vi "Update Registry.vi"() -> ()   [LabVIEW 2014]
uses:
  TypeDef/state.ctl
  TypeDef/Qmessage.ctl
  <vilib>/Utility/config.llb/Read Key (Path).vi
  <vilib>/Utility/file.llb/Read From Spreadsheet File (string).vi
  <vilib>/Utility/config.llb/Write Key (Path).vi
  <vilib>/Utility/config.llb/Read Key (String).vi
  <vilib>/Utility/config.llb/NI_LVConfig.lvlib
panel:
  out "Internal State":T1
  out "Date":string
  out "Time":string
  out "Status bar":string
  in  "Build New Config":bool
  in  "Tab Control":T2(tab)
  in  "Changed?":bool[](array[boolean])
  in  "Current Configuration":string[](array[string])
  in  "Component Name":string[](array[string])
  in  "New Configuration":string[](array[string])
  in  "Changed? 2":bool[](array[boolean])
  in  "Current Configuration 2":string[](array[string])
  in  "Component Name 2":string[](array[string])
  in  "New Configuration 2":string[](array[string])
  in  "Changed? 3":bool[](array[boolean])
  in  "Current Configuration 3":string[](array[string])
  in  "Component Name 3":string[](array[string])
  in  "New Configuration 3":string[](array[string])
  in  "Changed? 4":bool[](array[boolean])
  in  "Current Configuration 4":string[](array[string])
  in  "Component Name 4":string[](array[string])
  in  "New Configuration 4":string[](array[string])
  in  "Changed? 5":bool[](array[boolean])
  in  "Current Configuration 5":string[](array[string])
  in  "Component Name 5":string[](array[string])
  in  "New Configuration 5":string[](array[string])
  in  "Changed? 6":bool[](array[boolean])
  in  "Current Configuration 6":string[](array[string])
  in  "Component Name 6":string[](array[string])
  in  "New Configuration 6":string[](array[string])
  in  "Changed? 7":bool[](array[boolean])
  in  "Current Configuration 7":string[](array[string])
  in  "Component Name 7":string[](array[string])
  in  "New Configuration 7":string[](array[string])
  in  "Changed? 8":bool[](array[boolean])
  in  "Current Configuration 8":string[](array[string])
  in  "Component Name 8":string[](array[string])
  in  "New Configuration 8":string[](array[string])
  in  "Changed? 9":bool[](array[boolean])
  in  "Current Configuration 9":string[](array[string])
  in  "Component Name 9":string[](array[string])
  in  "New Configuration 9":string[](array[string])
  in  "Changed? 10":bool[](array[boolean])
  in  "Current Configuration 10":string[](array[string])
  in  "Component Name 10":string[](array[string])
  in  "New Configuration 10":string[](array[string])
  out "ini file path":path
  in  "variation sheet":path caption="Variation Sheet (*.ini)"
  in  "Push":bool
  in  "Help Button":bool
  in  "Run":bool
  in  "Initialize":bool
  in  "Register":bool
  in  "Add comment":bool
  in  "View":bool
  in  "tdms path":path caption="Variation Registry (*.tdms)"
  in  "Config Path":path caption="Config File (*.csv)"
  in  "Exit":bool
  # "Update Registry"
  # "New Configuration"
  # "Component Name"
  # "Current Configuration"
  # "New Configuration"
  # "Component Name"
  # "Current Configuration"
  # "New Configuration"
  # "Component Name"
  # "Current Configuration"
  # "New Configuration"
  # "Component Name"
  # "Current Configuration"
  # "New Configuration"
  # "Component Name"
  # "Current Configuration"
  # "New Configuration"
  # "Component Name"
  # "Current Configuration"
  # "New Configuration"
  # "Component Name"
  # "Current Configuration"
  # "New Configuration"
  # "Component Name"
  # "Current Configuration"
  # "New Configuration"
  # "Component Name"
  # "Current Configuration"
  # "New Configuration"
  # "Component Name"
  # "Current Configuration"
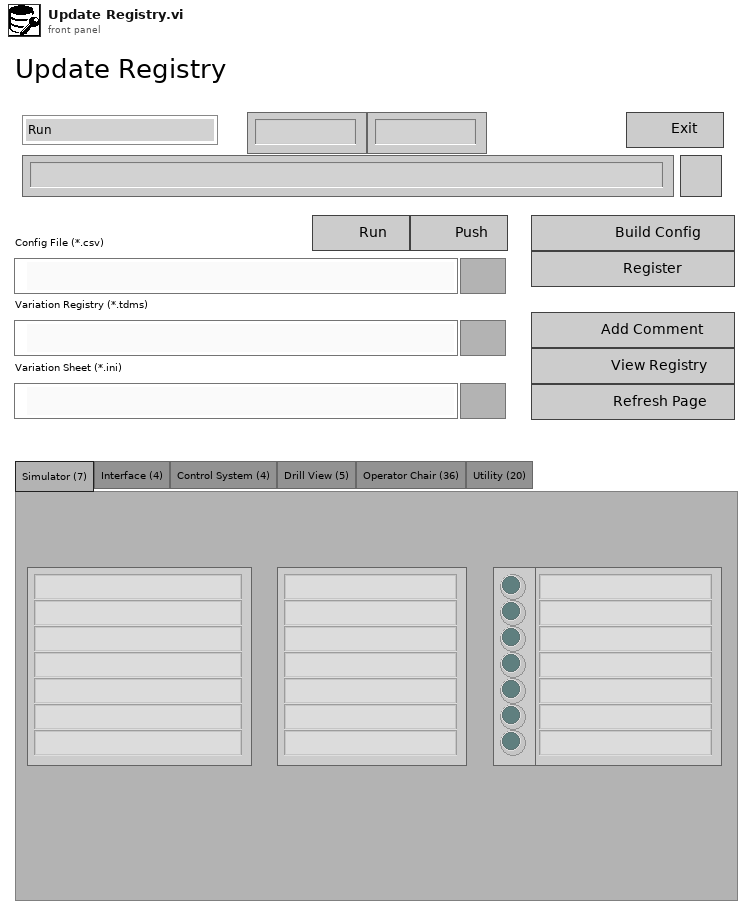
[diagram p1: front panel]
types:
  T1 = typedef "state.ctl" = enum16{"Run", "Initialize 1", "Initialize 2", "Read config file", "Read TDMS", "Config file Error", "Idle", "Update Comp Names", "Update Current Versions", "Make new configuration", "Register Change", "View Registry", "Add Comment", "No New Update", "Check current versions", "Read ini file", "Write ini file", "Read Variation Sheet", "Search and write current versions", "Close", "Update New Config", "Check ini file"}
  T2 = enum32{"Page 1", "Page 2", "Page 3", "Page 4", "Page 5", "Page 6", "Page 7", "Page 8", "Page 9", "Page 10"}
  T3 = cluster{"Folder Path containing version information":path, "File name (including .ini)":path, "Section":string}
  T4 = typedef "Qmessage.ctl" = cluster{"state":T1, "data":variant}
  T5 = cluster{"path":path, "This VI":refnum<vi>, "Level of Application":u8}
  T6 = enum32{"invalid app kind", "Development System", "Run Time System", "Student Edition", "Embedded LabVIEW", "Evaluation", "Custom"}
  T7 = cluster{"Current Version":string[], "Comp Name":string[]}
  T8 = enum8{"Enabled", "Disabled", "Disabled and Grayed Out"}
  T9 = typedef "NI_LVConfig.lvlib/Config Data RefNum.ctl" = refnum<k1>
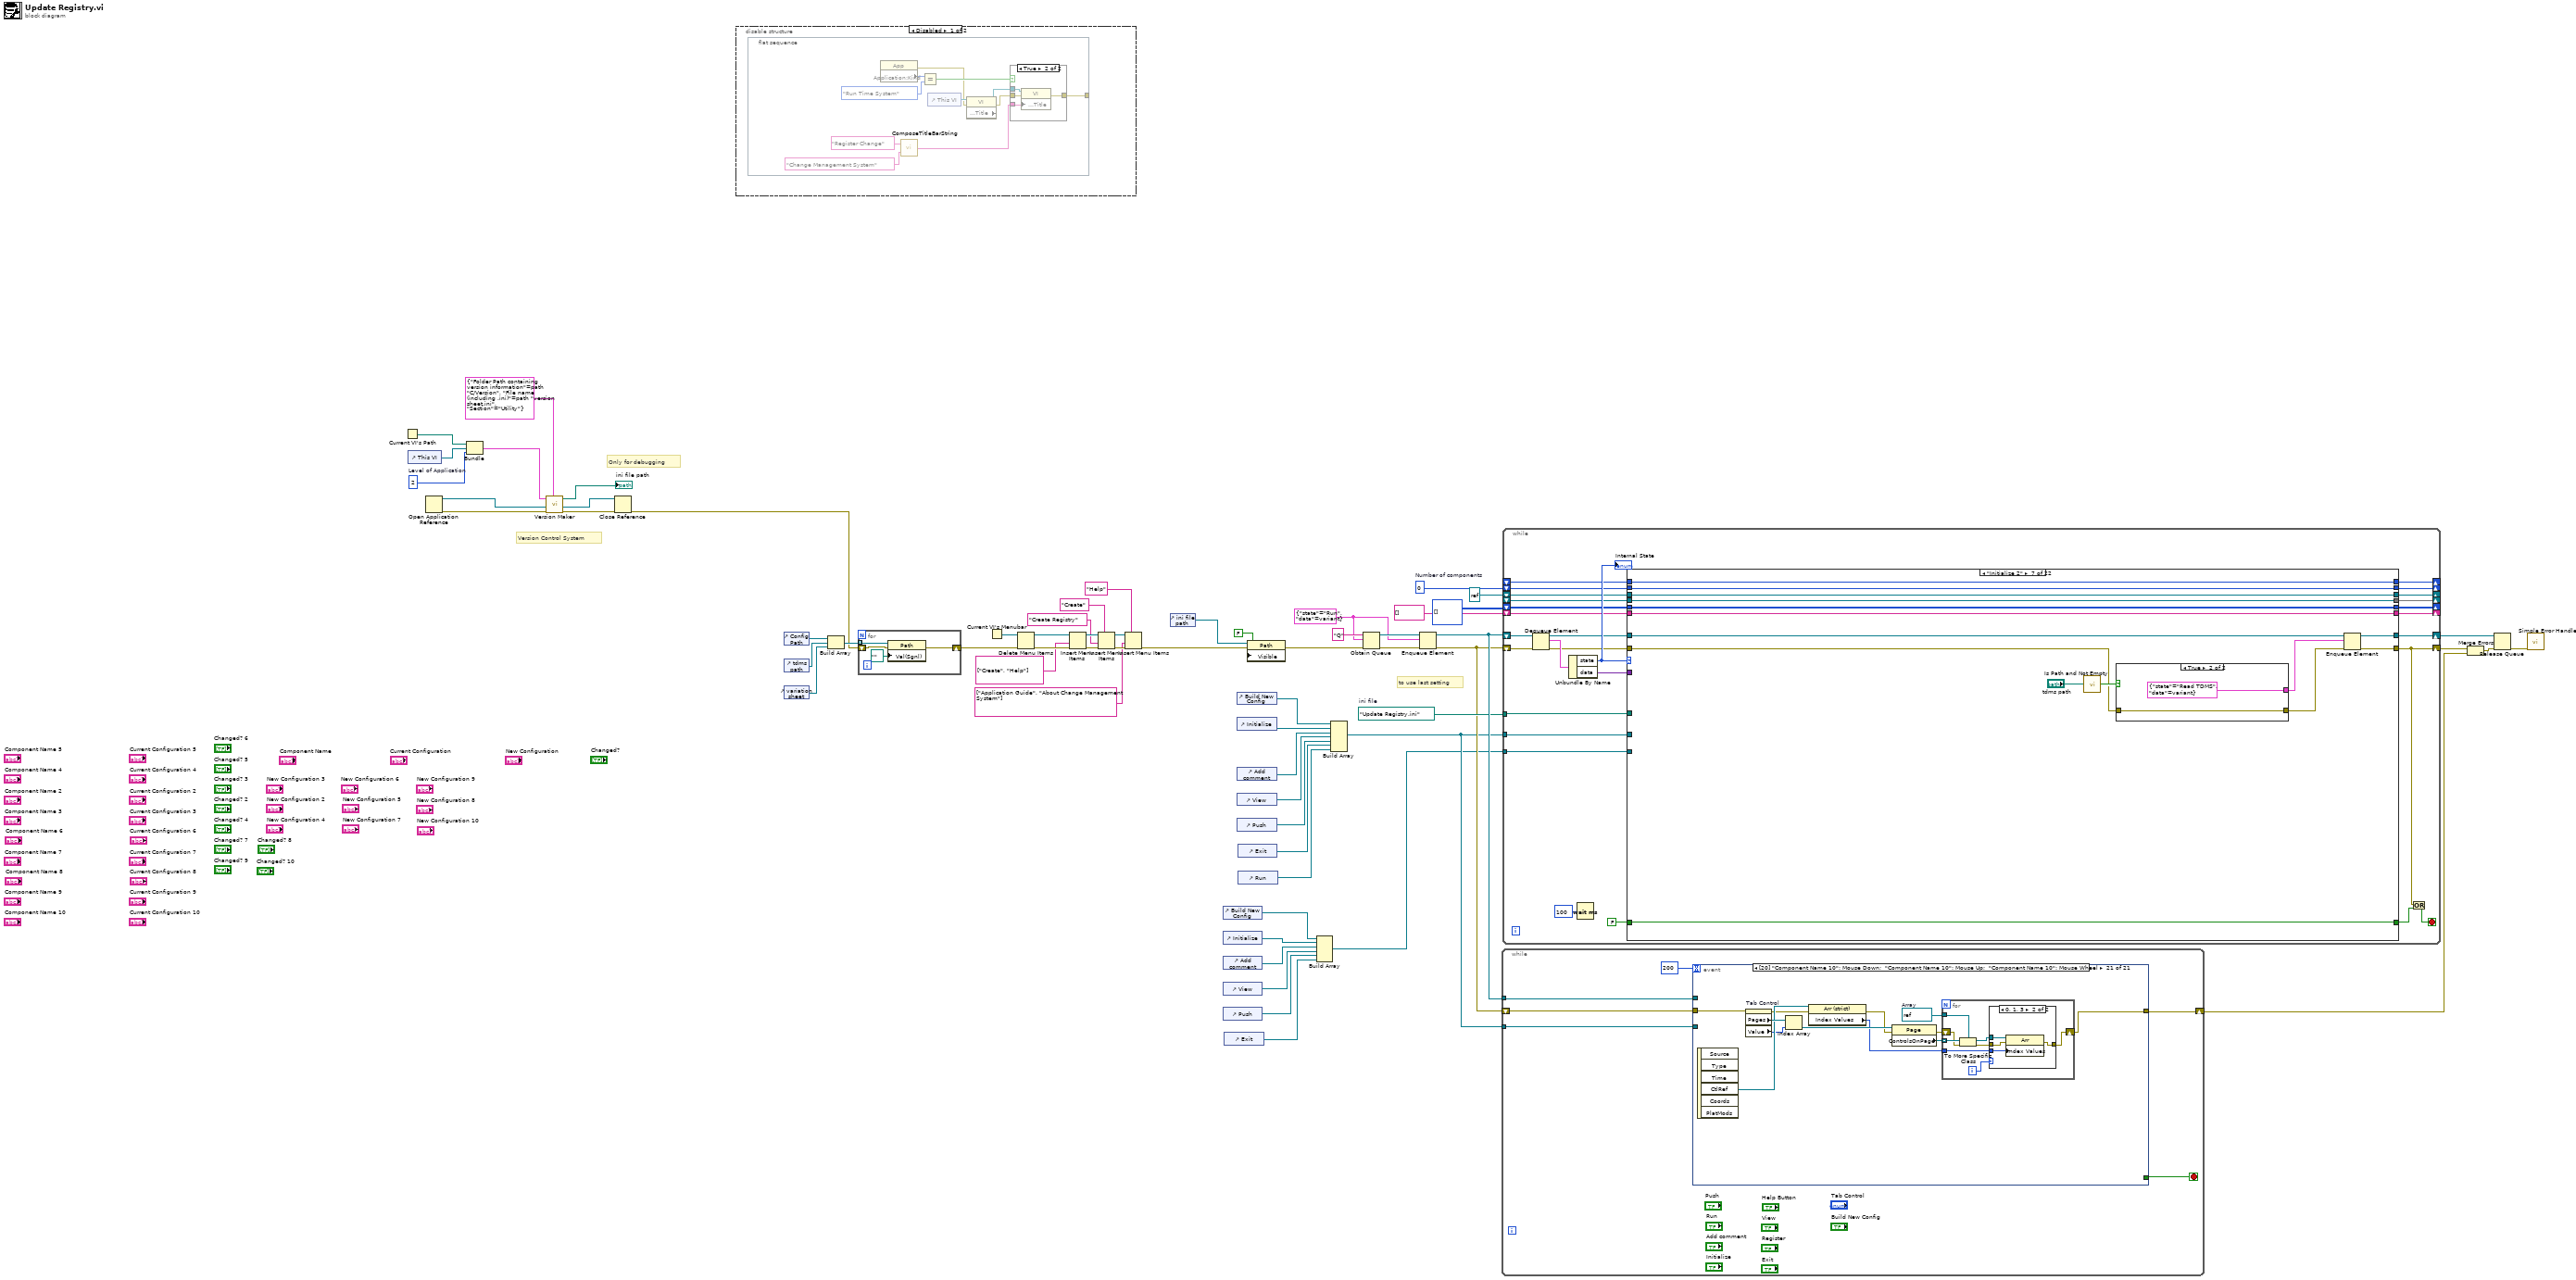
[diagram p0: block diagram]
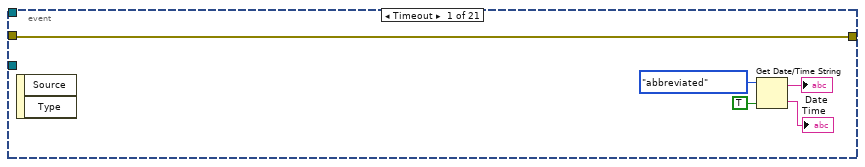
[diagram p4: hidden frame]
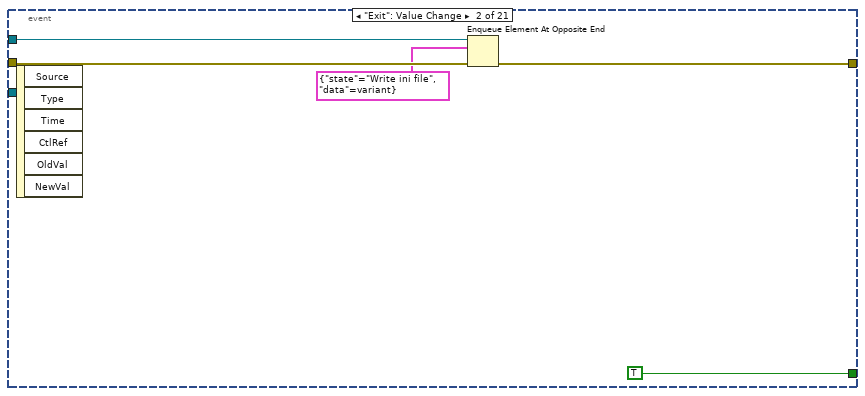
[diagram p5: hidden frame]
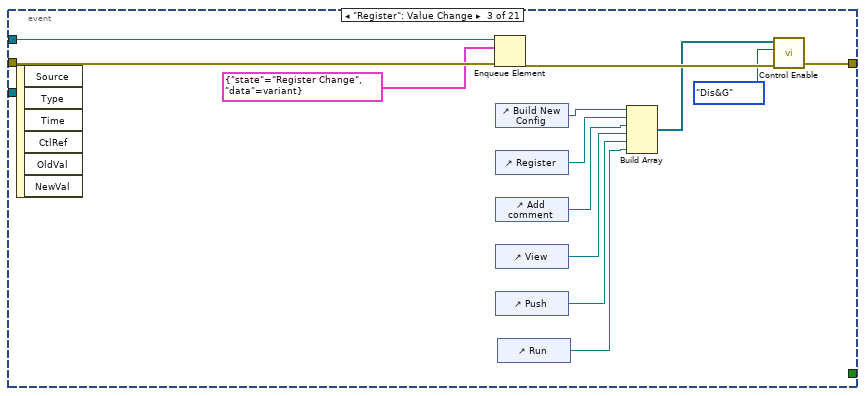
[diagram p6: hidden frame]
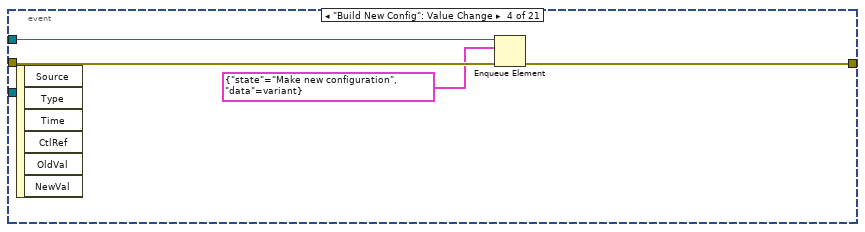
[diagram p7: hidden frame]
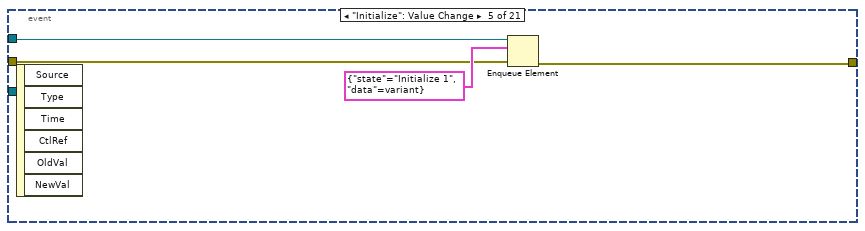
[diagram p8: hidden frame]
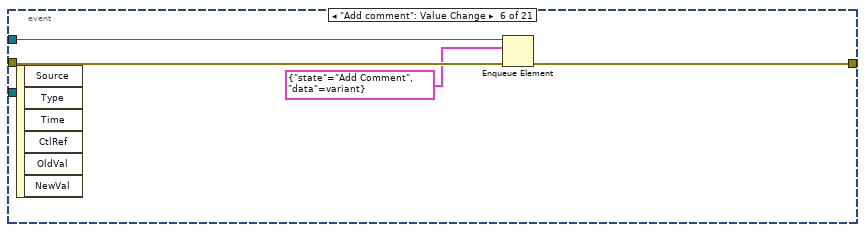
[diagram p9: hidden frame]
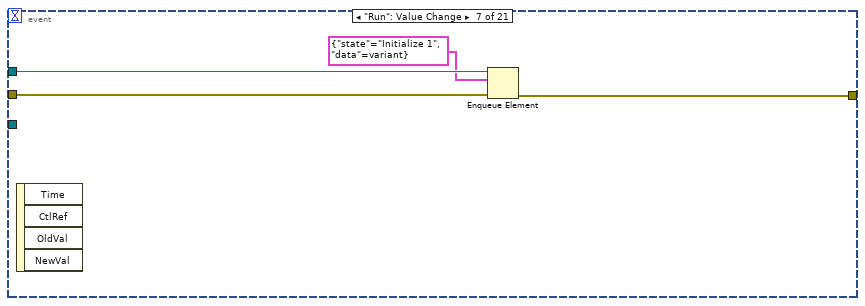
[diagram p10: hidden frame]
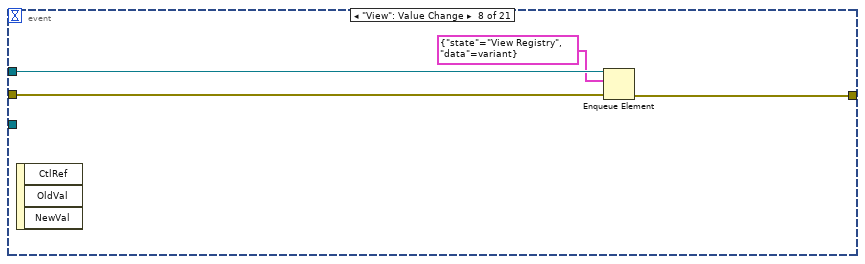
[diagram p11: hidden frame]
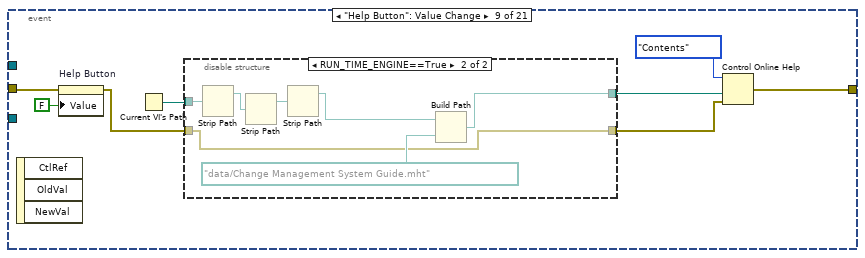
[diagram p12: hidden frame]
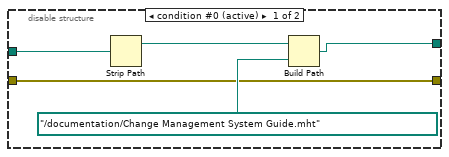
[diagram p13: hidden frame]
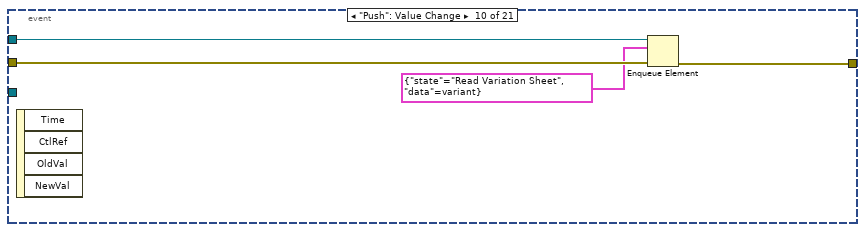
[diagram p14: hidden frame]
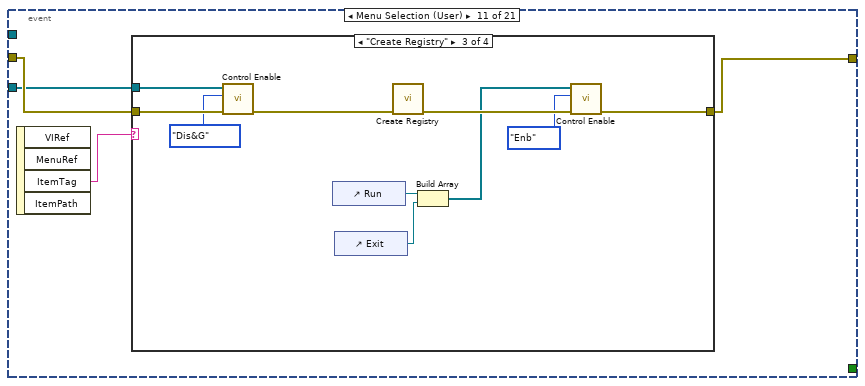
[diagram p15: hidden frame]
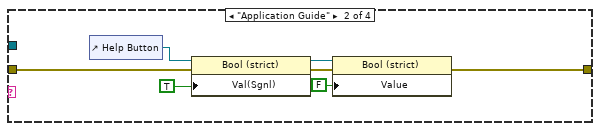
[diagram p17: hidden frame]
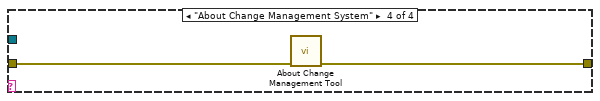
[diagram p18: hidden frame]
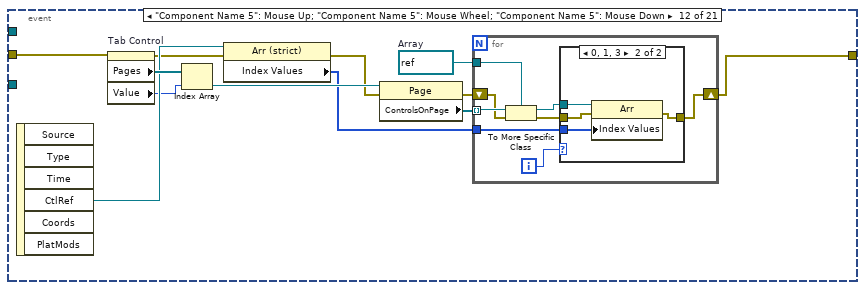
[diagram p19: hidden frame]
diagram:
  w44 = u8 2  # Level of Application
  w55 = path "Update Registry.ini"  # ini file
  w59 = 0  # Number of components
  w28 = T4 {"state"=enum."Run", "data"=variant} ("Cluster")
  # "to use last setting"
  # "Only for debugging"
  # "Version Control System"
  n1 = Current VI's Path() -> (path=w42:path)
  n2 = control-ref of="This VI"() -> (w43:refnum<vi>)
  n3 = Open Application Reference() -> (0:w54:errorcluster, 3:w50:refnum<vi>)  [unwired: 4 in]
  n4 = Bundle("path"=w42, "This VI"=w43, "Level of Application"=w44) -> (w45:T5)  [unwired: 1 in]
  n5 = call "Version Maker.vi"("Version Sheet Cluster"=T3 {"Folder Path containing version information"=path "C:/Version", "File name (including .ini)"=path "version sheet.ini", "Section"="Utility"}, "Error In"=w54, "Open Application Reference in"=w50, "VI Information"=w45) -> ("Error Out"=w53:errorcluster, "Open Application Reference out"=w49:refnum<vi>, "Standard Config Path"=→"ini file path":path)  [unwired: 4 in, 1 out]
  n6 = Close Reference(reference=w49, error in (no error)=w53) -> (error out=w22:errorcluster)
  n7 = disable-structure shown="Disabled" {
    frame Disabled {
      n8 = flat-sequence {
        tunnel: [w64] -> _
        frame #0 {
          n9 = property on="Property Node" class="App"() -> (error out=w66:errorcluster, "Application:Kind"=w72:T6)  [unwired: 2 in, 1 out]
          n10 = call "ComposeTitleBarString.vi"("ProjectName"="Change Management System" ("Application"), "Application"="Register Change") -> ("TitleBar"=w74:string)
          n11 = Equal?(x=w72, y=T6."Run Time System" ("Applikation:Typ")) -> (x = y?=w73:bool)
          n12 = control-ref of="This VI"() -> (w70:refnum<vi>)
          n13 = property on="Property Node" class="VI" props=["Front Panel.Title"](reference=w70, error in=w66) -> (reference out=w69:refnum<vi>, error out=w65:errorcluster)  [unwired: 1 out]
          n14 = case shown="True" w73 {
            tunnel: w74 -> [_ w79]
            tunnel: w69 -> [_ w78]
            tunnel: w65 -> [w75 w77]
            tunnel: [w75 w76] -> w64
            frame False {
            }
            frame True {
              n15 = property class="VI"(reference=w78, error in=w77, "Front Panel.Title"=w79) -> (error out=w76:errorcluster)  [unwired: 1 out]
            }
          }
        }
      }
    }
    frame Enabled {
    }
  }
  n16 = control-ref of="Config Path"() -> (w26:refnum<vi>)
  n17 = control-ref of="tdms path"() -> (w25:refnum<vi>)
  n18 = control-ref of="variation sheet"() -> (w24:refnum<vi>)
  n19 = Build Array(w26, w25, w24) -> (w23:refnum<vi>[])
  n20 = for {
    tunnel: w23 -> [w83] mode=indexing
    shift-right: [w81] -> w21
    shift-left: w22 -> [w80]
    n21 = property class="Path"(reference=w83, error in=w80, "Val(Sgnl)"=path "" ("Value (Signaling)")) -> (error out=w81:errorcluster)  [unwired: 1 out]
  }
  n22 = Current VI's Menubar() -> (w41:refnum<k9>)
  n23 = Delete Menu Items(6:w21, 9:w41) -> (0:w40:errorcluster, 3:w39:refnum<k9>)  [unwired: 2 in]
  n24 = Insert Menu Items(6:w40, 7:string[] ["Create", "Help"] ("item tags"), 9:w39) -> (0:w35:errorcluster, 3:w37:refnum<k9>)  [unwired: 3 in, 1 out]
  n25 = Insert Menu Items(5:"Create", 6:w35, 7:"Create Registry", 9:w37) -> (0:w34:errorcluster, 3:w33:refnum<k9>)  [unwired: 2 in, 1 out]
  n26 = Insert Menu Items(5:"Help", 6:w34, 7:string[] ["Application Guide", "About Change Management System"] ("item tags"), 9:w33) -> (0:w27:errorcluster)  [unwired: 2 in, 2 out]
  n27 = control-ref of="ini file path"() -> (w47:refnum<vi>)
  n28 = control-ref of="Build New Config"() -> (w2:refnum<vi>)
  n29 = control-ref of="Initialize"() -> (w3:refnum<vi>)
  n30 = control-ref of="Add comment"() -> (w5:refnum<vi>)
  n31 = control-ref of="View"() -> (w6:refnum<vi>)
  n32 = control-ref of="Push"() -> (w7:refnum<vi>)
  n33 = control-ref of="Exit"() -> (w4:refnum<vi>)
  n34 = control-ref of="Build New Config"() -> (w8:refnum<vi>)
  n35 = control-ref of="Initialize"() -> (w9:refnum<vi>)
  n36 = control-ref of="Add comment"() -> (w15:refnum<vi>)
  n37 = control-ref of="View"() -> (w14:refnum<vi>)
  n38 = control-ref of="Push"() -> (w13:refnum<vi>)
  n39 = control-ref of="Exit"() -> (w12:refnum<vi>)
  n40 = control-ref of="Run"() -> (w11:refnum<vi>)
  n41 = property class="Path"(reference=w47, error in=w27, "Visible"=FALSE) -> (error out=w48:errorcluster)  [unwired: 1 out]
  n42 = Build Array(w2, w3, w5, w6, w7, w4) -> (w1:refnum<vi>[])
  n43 = Build Array(w8, w9, w15, w14, w13, w12, w11) -> (w10:refnum<vi>[])
  n44 = Obtain Queue(name (unnamed)="Q", element data type=w28, error in (no error)=w48) -> (queue out=w63:refnum<queue>, error out=w58:errorcluster)  [unwired: 2 in, 1 out]
  n45 = Enqueue Element(queue=w63, element=w28, error in (no error)=w58) -> (queue out=w61:refnum<queue>, error out=w29:errorcluster)  [unwired: 1 in, 1 out]
  n46 = while {
    tunnel: w61 -> [w89]
    tunnel: w10 -> [w86]
    shift-right: [w85] -> w18
    shift-left: w29 -> [w87]
    stop <- w88 stop-if-true
    n47 = event shown="[20] \"Component Name 10\": Mouse Down;  \"Component Name 10\": Mouse Up;  \"Component Name 10\": Mouse Wheel" {
      selector: _ -> [_ _ _ _ _ _ _ _ _ _ _ _ _ _ _ _ _ _ _ _ _]
      dyn-events: _ -> [_ _ _ _ _ _ _ _ _ _ _ _ _ _ _ _ _ _ _ _ _]
      timeout: u32 200 ("milliseconds to wait") -> [_ _ _ _ _ _ _ _ _ _ _ _ _ _ _ _ _ _ _ _ _]
      tunnel: w89 -> [_ w99 w112 w116 w120 w124 w128 w132 _ w156 _ _ _ _ _ _ _ _ _ _ _]
      tunnel: [_ TRUE _ _ _ _ _ _ _ _ _ _ _ _ _ _ _ _ _ _ _] -> w88
      tunnel: [w90 w97 w109 w113 w119 w123 w127 w131 w139 w155 w158 w182 w207 w232 w257 w282 w307 w332 w357 w382 w407] -> w85
      tunnel: w87 -> [w90 w96 w111 w115 w117 w122 w126 w130 w135 w154 w159 w190 w215 w240 w265 w290 w315 w340 w365 w390 w415]
      tunnel: w86 -> [_ _ _ _ _ _ _ _ _ _ w157 _ _ _ _ _ _ _ _ _ _]
      event Timeout {
        n48 = event-data() -> ()  [unwired: 1 in, 2 out]
        n49 = Get Date/Time String(date format (0)=enum16{"short", "long", "abbreviated"}."abbreviated", want seconds? (F)=TRUE) -> (date string=→"Date":string, time string=→"Time":string)  [unwired: 1 in]
      }
      event "Exit": Value Change {
        n50 = event-data() -> ()  [unwired: 1 in, 6 out]
        n51 = Enqueue Element At Opposite End(queue=w99, element=T4 {"state"=enum."Write ini file", "data"=variant} ("Cluster"), error in (no error)=w96) -> (error out=w97:errorcluster)  [unwired: 1 in, 2 out]
      }
      event "Register": Value Change {
        n52 = event-data() -> ()  [unwired: 1 in, 6 out]
        n53 = Enqueue Element(queue=w112, element=T4 {"state"=enum."Register Change", "data"=variant} ("Cluster"), error in (no error)=w111) -> (error out=w108:errorcluster)  [unwired: 1 in, 2 out]
        n54 = control-ref of="Build New Config"() -> (w101:refnum<vi>)
        n55 = control-ref of="Register"() -> (w102:refnum<vi>)
        n56 = control-ref of="Add comment"() -> (w103:refnum<vi>)
        n57 = control-ref of="View"() -> (w104:refnum<vi>)
        n58 = control-ref of="Push"() -> (w105:refnum<vi>)
        n59 = control-ref of="Run"() -> (w106:refnum<vi>)
        n60 = Build Array(w101, w102, w103, w104, w105, w106) -> (w100:refnum<vi>[])
        n61 = call "Control Enable.vi"("error in (no error)"=w108, "Enum"=enum16{"Enb", "Dis", "Dis&G"}."Dis&G", "Reference Array"=w100) -> ("error out"=w109:errorcluster)  [unwired: 8 in]
      }
      event "Build New Config": Value Change {
        n62 = event-data() -> ()  [unwired: 1 in, 6 out]
        n63 = Enqueue Element(queue=w116, element=T4 {"state"=enum."Make new configuration", "data"=variant} ("Cluster"), error in (no error)=w115) -> (error out=w113:errorcluster)  [unwired: 1 in, 2 out]
      }
      event "Initialize": Value Change {
        n64 = event-data() -> ()  [unwired: 1 in, 6 out]
        n65 = Enqueue Element(queue=w120, element=T4 {"state"=enum."Initialize 1", "data"=variant} ("Cluster"), error in (no error)=w117) -> (error out=w119:errorcluster)  [unwired: 1 in, 2 out]
      }
      event "Add comment": Value Change {
        n66 = event-data() -> ()  [unwired: 1 in, 6 out]
        n67 = Enqueue Element(queue=w124, element=T4 {"state"=enum."Add Comment", "data"=variant} ("Cluster"), error in (no error)=w122) -> (error out=w123:errorcluster)  [unwired: 1 in, 2 out]
      }
      event "Run": Value Change {
        n68 = event-data() -> ()  [unwired: 1 in, 4 out]
        n69 = Enqueue Element(queue=w128, element=T4 {"state"=enum."Initialize 1", "data"=variant} ("Cluster"), error in (no error)=w126) -> (error out=w127:errorcluster)  [unwired: 1 in, 2 out]
      }
      event "View": Value Change {
        n70 = event-data() -> ()  [unwired: 1 in, 3 out]
        n71 = Enqueue Element(queue=w132, element=T4 {"state"=enum."View Registry", "data"=variant} ("Cluster"), error in (no error)=w130) -> (error out=w131:errorcluster)  [unwired: 1 in, 2 out]
      }
      event "Help Button": Value Change {
        n72 = event-data() -> ()  [unwired: 1 in, 3 out]
        n73 = property on="Help Button" class="Bool (strict)"(error in=w135, "Value"=FALSE ("Help Button")) -> (error out=w134:errorcluster)  [unwired: 1 in, 1 out]
        n74 = Current VI's Path() -> (path=w138:path)
        n75 = disable-structure shown="RUN_TIME_ENGINE==True" {
          disable-tunnel: w138 -> [w145 w152]
          disable-tunnel: [w142 w148] -> w137
          disable-tunnel: w134 -> [w141 w146]
          disable-tunnel: [w141 w146] -> w133
          frame condition #0 (active) {
            n76 = Strip Path(path=w145) -> (stripped path=w144:path)  [unwired: 1 out]
            n77 = Build Path(base path=w144, name or relative path=path "../documentation/Change Management System Guide.mht") -> (appended path=w142:path)
          }
          frame condition #1 {
            n78 = Strip Path(path=w152) -> (stripped path=w151:path)  [unwired: 1 out]
            n79 = Strip Path(path=w151) -> (stripped path=w150:path)  [unwired: 1 out]
            n80 = Strip Path(path=w150) -> (stripped path=w147:path)  [unwired: 1 out]
            n81 = Build Path(base path=w147, name or relative path=path "data/Change Management System Guide.mht") -> (appended path=w148:path)
          }
        }
        n82 = Control Online Help(1:w133, 2:w137, 4:enum16{"Contents", "Key", "Close"}."Contents" ("Operation")) -> (0:w139:errorcluster)  [unwired: 1 in]
      }
      event "Push": Value Change {
        n83 = event-data() -> ()  [unwired: 1 in, 4 out]
        n84 = Enqueue Element(queue=w156, element=T4 {"state"=enum."Read Variation Sheet", "data"=variant} ("Cluster"), error in (no error)=w154) -> (error out=w155:errorcluster)  [unwired: 1 in, 2 out]
      }
      event Menu Selection (User) {
        n85 = event-data() -> ("ItemTag"=w160:string)  [unwired: 1 in, 3 out]
        n86 = case shown="\"Create Registry\"" w160 {
          tunnel: w159 -> [w161 w163 w176 w180]
          tunnel: [w161 w162 w173 w179] -> w158
          tunnel: w157 -> [_ _ w172 _]
          frame "default", Default {
          }
          frame "Application Guide" {
            n87 = control-ref of="Help Button"() -> (w168:refnum<vi>)
            n88 = property class="Bool (strict)"(reference=w168, error in=w163, "Val(Sgnl)"=TRUE) -> (reference out=w166:refnum<vi>, error out=w165:errorcluster)
            n89 = property class="Bool (strict)"(reference=w166, error in=w165, "Value"=FALSE ("Value (Signaling)")) -> (error out=w162:errorcluster)  [unwired: 1 out]
          }
          frame "Create Registry" {
            n90 = call "Control Enable.vi"("error in (no error)"=w176, "Enum"=enum16{"Enb", "Dis", "Dis&G"}."Dis&G", "Reference Array"=w172) -> ("error out"=w175:errorcluster)  [unwired: 8 in]
            n91 = control-ref of="Run"() -> (w177:refnum<vi>)
            n92 = control-ref of="Exit"() -> (w178:refnum<vi>)
            n93 = call "Create Registry.vi"("Error In"=w175) -> ("Error Out"=w174:errorcluster)  [unwired: 10 in]
            n94 = Build Array(w177, w178) -> (w170:refnum<vi>[])
            n95 = call "Control Enable.vi"("error in (no error)"=w174, "Enum"=enum16{"Enb", "Dis", "Dis&G"}."Enb", "Reference Array"=w170) -> ("error out"=w173:errorcluster)  [unwired: 8 in]
          }
          frame "About Change Management System" {
            n96 = call "About Change Management Tool.vi"("Error In"=w180) -> ("Error Out"=w179:errorcluster)  [unwired: 10 in]
          }
        }
      }
      event "Component Name 5": Mouse Up; "Component Name 5": Mouse Wheel; "Component Name 5": Mouse Down {
        w191 = refnum<vi> refnum  # Array
        n97 = event-data() -> ("CtlRef"=w188:refnum<vi>)  [unwired: 1 in, 5 out]
        n98 = property on="Tab Control" class="TabCtl (strict)"(error in=w190) -> (error out=w187:errorcluster, "Pages"=w189:refnum<vi>[], "Value"=w184:T2)  [unwired: 1 in, 1 out]
        n99 = Index Array(array=w189, index=w184) -> (element=w186:refnum<vi>)
        n100 = property class="Arr (strict)"(reference=w188, error in=w187) -> (error out=w185:errorcluster, "Index Values"=w181:u32[])  [unwired: 1 out]
        n101 = property class="Page"(reference=w186, error in=w185) -> (error out=w183:errorcluster, "ControlsOnPage"=w192:refnum<vi>[])  [unwired: 1 out]
        n102 = for {
          tunnel: w192 -> [w198] mode=indexing
          tunnel: w191 -> [w197]
          tunnel: w181 -> [w196]
          shift-right: [w193] -> w182
          shift-left: w183 -> [w195]
          i -> [w200]
          n103 = To More Specific Class(target class=w197, reference=w198, error in=w195) -> (specific class reference=w199:refnum<vi>, error out=w194:errorcluster)
          n104 = case shown="0, 1, 3" w200 {
            tunnel: w199 -> [_ w205]
            tunnel: w196 -> [_ w204]
            tunnel: w194 -> [w201 w203]
            tunnel: [w201 w202] -> w193
            frame 2, Default {
            }
            frame 0, 1, 3 {
              n105 = property class="Arr"(reference=w205, error in=w203, "Index Values"=w204) -> (error out=w202:errorcluster)  [unwired: 1 out]
            }
          }
        }
      }
      event "Component Name": Mouse Wheel; "Component Name": Mouse Down; "Component Name": Mouse Up {
        w216 = refnum<vi> refnum  # Array
        n106 = event-data() -> ("CtlRef"=w213:refnum<vi>)  [unwired: 1 in, 5 out]
        n107 = property on="Tab Control" class="TabCtl (strict)"(error in=w215) -> (error out=w212:errorcluster, "Pages"=w214:refnum<vi>[], "Value"=w209:T2)  [unwired: 1 in, 1 out]
        n108 = Index Array(array=w214, index=w209) -> (element=w211:refnum<vi>)
        n109 = property class="Arr (strict)"(reference=w213, error in=w212) -> (error out=w210:errorcluster, "Index Values"=w206:u32[])  [unwired: 1 out]
        n110 = property class="Page"(reference=w211, error in=w210) -> (error out=w208:errorcluster, "ControlsOnPage"=w217:refnum<vi>[])  [unwired: 1 out]
        n111 = for {
          tunnel: w217 -> [w223] mode=indexing
          tunnel: w216 -> [w222]
          tunnel: w206 -> [w221]
          shift-right: [w218] -> w207
          shift-left: w208 -> [w220]
          i -> [w225]
          n112 = To More Specific Class(target class=w222, reference=w223, error in=w220) -> (specific class reference=w224:refnum<vi>, error out=w219:errorcluster)
          n113 = case shown="0, 1, 3" w225 {
            tunnel: w224 -> [_ w230]
            tunnel: w221 -> [_ w229]
            tunnel: w219 -> [w226 w228]
            tunnel: [w226 w227] -> w218
            frame 2, Default {
            }
            frame 0, 1, 3 {
              n114 = property class="Arr"(reference=w230, error in=w228, "Index Values"=w229) -> (error out=w227:errorcluster)  [unwired: 1 out]
            }
          }
        }
      }
      event "Component Name 2": Mouse Wheel; "Component Name 2": Mouse Down; "Component Name 2": Mouse Up {
        w241 = refnum<vi> refnum  # Array
        n115 = event-data() -> ("CtlRef"=w238:refnum<vi>)  [unwired: 1 in, 5 out]
        n116 = property on="Tab Control" class="TabCtl (strict)"(error in=w240) -> (error out=w237:errorcluster, "Pages"=w239:refnum<vi>[], "Value"=w234:T2)  [unwired: 1 in, 1 out]
        n117 = Index Array(array=w239, index=w234) -> (element=w236:refnum<vi>)
        n118 = property class="Arr (strict)"(reference=w238, error in=w237) -> (error out=w235:errorcluster, "Index Values"=w231:u32[])  [unwired: 1 out]
        n119 = property class="Page"(reference=w236, error in=w235) -> (error out=w233:errorcluster, "ControlsOnPage"=w242:refnum<vi>[])  [unwired: 1 out]
        n120 = for {
          tunnel: w242 -> [w248] mode=indexing
          tunnel: w241 -> [w247]
          tunnel: w231 -> [w246]
          shift-right: [w243] -> w232
          shift-left: w233 -> [w245]
          i -> [w250]
          n121 = To More Specific Class(target class=w247, reference=w248, error in=w245) -> (specific class reference=w249:refnum<vi>, error out=w244:errorcluster)
          n122 = case shown="0, 1, 3" w250 {
            tunnel: w249 -> [_ w255]
            tunnel: w246 -> [_ w254]
            tunnel: w244 -> [w251 w253]
            tunnel: [w251 w252] -> w243
            frame 2, Default {
            }
            frame 0, 1, 3 {
              n123 = property class="Arr"(reference=w255, error in=w253, "Index Values"=w254) -> (error out=w252:errorcluster)  [unwired: 1 out]
            }
          }
        }
      }
      event "Component Name 3": Mouse Wheel; "Component Name 3": Mouse Up; "Component Name 3": Mouse Down {
        w266 = refnum<vi> refnum  # Array
        n124 = event-data() -> ("CtlRef"=w263:refnum<vi>)  [unwired: 1 in, 5 out]
        n125 = property on="Tab Control" class="TabCtl (strict)"(error in=w265) -> (error out=w262:errorcluster, "Pages"=w264:refnum<vi>[], "Value"=w259:T2)  [unwired: 1 in, 1 out]
        n126 = Index Array(array=w264, index=w259) -> (element=w261:refnum<vi>)
        n127 = property class="Arr (strict)"(reference=w263, error in=w262) -> (error out=w260:errorcluster, "Index Values"=w256:u32[])  [unwired: 1 out]
        n128 = property class="Page"(reference=w261, error in=w260) -> (error out=w258:errorcluster, "ControlsOnPage"=w267:refnum<vi>[])  [unwired: 1 out]
        n129 = for {
          tunnel: w267 -> [w273] mode=indexing
          tunnel: w266 -> [w272]
          tunnel: w256 -> [w271]
          shift-right: [w268] -> w257
          shift-left: w258 -> [w270]
          i -> [w275]
          n130 = To More Specific Class(target class=w272, reference=w273, error in=w270) -> (specific class reference=w274:refnum<vi>, error out=w269:errorcluster)
          n131 = case shown="0, 1, 3" w275 {
            tunnel: w274 -> [_ w280]
            tunnel: w271 -> [_ w279]
            tunnel: w269 -> [w276 w278]
            tunnel: [w276 w277] -> w268
            frame 2, Default {
            }
            frame 0, 1, 3 {
              n132 = property class="Arr"(reference=w280, error in=w278, "Index Values"=w279) -> (error out=w277:errorcluster)  [unwired: 1 out]
            }
          }
        }
      }
      event "Component Name 4": Mouse Wheel; "Component Name 4": Mouse Up; "Component Name 4": Mouse Down {
        w291 = refnum<vi> refnum  # Array
        n133 = event-data() -> ("CtlRef"=w288:refnum<vi>)  [unwired: 1 in, 5 out]
        n134 = property on="Tab Control" class="TabCtl (strict)"(error in=w290) -> (error out=w287:errorcluster, "Pages"=w289:refnum<vi>[], "Value"=w284:T2)  [unwired: 1 in, 1 out]
        n135 = Index Array(array=w289, index=w284) -> (element=w286:refnum<vi>)
        n136 = property class="Arr (strict)"(reference=w288, error in=w287) -> (error out=w285:errorcluster, "Index Values"=w281:u32[])  [unwired: 1 out]
        n137 = property class="Page"(reference=w286, error in=w285) -> (error out=w283:errorcluster, "ControlsOnPage"=w292:refnum<vi>[])  [unwired: 1 out]
        n138 = for {
          tunnel: w292 -> [w298] mode=indexing
          tunnel: w291 -> [w297]
          tunnel: w281 -> [w296]
          shift-right: [w293] -> w282
          shift-left: w283 -> [w295]
          i -> [w300]
          n139 = To More Specific Class(target class=w297, reference=w298, error in=w295) -> (specific class reference=w299:refnum<vi>, error out=w294:errorcluster)
          n140 = case shown="0, 1, 3" w300 {
            tunnel: w299 -> [_ w305]
            tunnel: w296 -> [_ w304]
            tunnel: w294 -> [w301 w303]
            tunnel: [w301 w302] -> w293
            frame 2, Default {
            }
            frame 0, 1, 3 {
              n141 = property class="Arr"(reference=w305, error in=w303, "Index Values"=w304) -> (error out=w302:errorcluster)  [unwired: 1 out]
            }
          }
        }
      }
      event "Component Name 6": Mouse Wheel; "Component Name 6": Mouse Up; "Component Name 6": Mouse Down {
        w316 = refnum<vi> refnum  # Array
        n142 = event-data() -> ("CtlRef"=w313:refnum<vi>)  [unwired: 1 in, 5 out]
        n143 = property on="Tab Control" class="TabCtl (strict)"(error in=w315) -> (error out=w312:errorcluster, "Pages"=w314:refnum<vi>[], "Value"=w309:T2)  [unwired: 1 in, 1 out]
        n144 = Index Array(array=w314, index=w309) -> (element=w311:refnum<vi>)
        n145 = property class="Arr (strict)"(reference=w313, error in=w312) -> (error out=w310:errorcluster, "Index Values"=w306:u32[])  [unwired: 1 out]
        n146 = property class="Page"(reference=w311, error in=w310) -> (error out=w308:errorcluster, "ControlsOnPage"=w317:refnum<vi>[])  [unwired: 1 out]
        n147 = for {
          tunnel: w317 -> [w323] mode=indexing
          tunnel: w316 -> [w322]
          tunnel: w306 -> [w321]
          shift-right: [w318] -> w307
          shift-left: w308 -> [w320]
          i -> [w325]
          n148 = To More Specific Class(target class=w322, reference=w323, error in=w320) -> (specific class reference=w324:refnum<vi>, error out=w319:errorcluster)
          n149 = case shown="0, 1, 3" w325 {
            tunnel: w324 -> [_ w330]
            tunnel: w321 -> [_ w329]
            tunnel: w319 -> [w326 w328]
            tunnel: [w326 w327] -> w318
            frame 2, Default {
            }
            frame 0, 1, 3 {
              n150 = property class="Arr"(reference=w330, error in=w328, "Index Values"=w329) -> (error out=w327:errorcluster)  [unwired: 1 out]
            }
          }
        }
      }
      event "Component Name 7": Mouse Wheel; "Component Name 7": Mouse Up; "Component Name 7": Mouse Down {
        w341 = refnum<vi> refnum  # Array
        n151 = event-data() -> ("CtlRef"=w338:refnum<vi>)  [unwired: 1 in, 5 out]
        n152 = property on="Tab Control" class="TabCtl (strict)"(error in=w340) -> (error out=w337:errorcluster, "Pages"=w339:refnum<vi>[], "Value"=w334:T2)  [unwired: 1 in, 1 out]
        n153 = Index Array(array=w339, index=w334) -> (element=w336:refnum<vi>)
        n154 = property class="Arr (strict)"(reference=w338, error in=w337) -> (error out=w335:errorcluster, "Index Values"=w331:u32[])  [unwired: 1 out]
        n155 = property class="Page"(reference=w336, error in=w335) -> (error out=w333:errorcluster, "ControlsOnPage"=w342:refnum<vi>[])  [unwired: 1 out]
        n156 = for {
          tunnel: w342 -> [w348] mode=indexing
          tunnel: w341 -> [w347]
          tunnel: w331 -> [w346]
          shift-right: [w343] -> w332
          shift-left: w333 -> [w345]
          i -> [w350]
          n157 = To More Specific Class(target class=w347, reference=w348, error in=w345) -> (specific class reference=w349:refnum<vi>, error out=w344:errorcluster)
          n158 = case shown="0, 1, 3" w350 {
            tunnel: w349 -> [_ w355]
            tunnel: w346 -> [_ w354]
            tunnel: w344 -> [w351 w353]
            tunnel: [w351 w352] -> w343
            frame 2, Default {
            }
            frame 0, 1, 3 {
              n159 = property class="Arr"(reference=w355, error in=w353, "Index Values"=w354) -> (error out=w352:errorcluster)  [unwired: 1 out]
            }
          }
        }
      }
      event "Component Name 8": Mouse Wheel; "Component Name 8": Mouse Down; "Component Name 8": Mouse Up {
        w366 = refnum<vi> refnum  # Array
        n160 = event-data() -> ("CtlRef"=w363:refnum<vi>)  [unwired: 1 in, 5 out]
        n161 = property on="Tab Control" class="TabCtl (strict)"(error in=w365) -> (error out=w362:errorcluster, "Pages"=w364:refnum<vi>[], "Value"=w359:T2)  [unwired: 1 in, 1 out]
        n162 = Index Array(array=w364, index=w359) -> (element=w361:refnum<vi>)
        n163 = property class="Arr (strict)"(reference=w363, error in=w362) -> (error out=w360:errorcluster, "Index Values"=w356:u32[])  [unwired: 1 out]
        n164 = property class="Page"(reference=w361, error in=w360) -> (error out=w358:errorcluster, "ControlsOnPage"=w367:refnum<vi>[])  [unwired: 1 out]
        n165 = for {
          tunnel: w367 -> [w373] mode=indexing
          tunnel: w366 -> [w372]
          tunnel: w356 -> [w371]
          shift-right: [w368] -> w357
          shift-left: w358 -> [w370]
          i -> [w375]
          n166 = To More Specific Class(target class=w372, reference=w373, error in=w370) -> (specific class reference=w374:refnum<vi>, error out=w369:errorcluster)
          n167 = case shown="0, 1, 3" w375 {
            tunnel: w374 -> [_ w380]
            tunnel: w371 -> [_ w379]
            tunnel: w369 -> [w376 w378]
            tunnel: [w376 w377] -> w368
            frame 2, Default {
            }
            frame 0, 1, 3 {
              n168 = property class="Arr"(reference=w380, error in=w378, "Index Values"=w379) -> (error out=w377:errorcluster)  [unwired: 1 out]
            }
          }
        }
      }
      event "Component Name 9": Mouse Wheel; "Component Name 9": Mouse Up; "Component Name 9": Mouse Down {
        w391 = refnum<vi> refnum  # Array
        n169 = event-data() -> ("CtlRef"=w388:refnum<vi>)  [unwired: 1 in, 5 out]
        n170 = property on="Tab Control" class="TabCtl (strict)"(error in=w390) -> (error out=w387:errorcluster, "Pages"=w389:refnum<vi>[], "Value"=w384:T2)  [unwired: 1 in, 1 out]
        n171 = Index Array(array=w389, index=w384) -> (element=w386:refnum<vi>)
        n172 = property class="Arr (strict)"(reference=w388, error in=w387) -> (error out=w385:errorcluster, "Index Values"=w381:u32[])  [unwired: 1 out]
        n173 = property class="Page"(reference=w386, error in=w385) -> (error out=w383:errorcluster, "ControlsOnPage"=w392:refnum<vi>[])  [unwired: 1 out]
        n174 = for {
          tunnel: w392 -> [w398] mode=indexing
          tunnel: w391 -> [w397]
          tunnel: w381 -> [w396]
          shift-right: [w393] -> w382
          shift-left: w383 -> [w395]
          i -> [w400]
          n175 = To More Specific Class(target class=w397, reference=w398, error in=w395) -> (specific class reference=w399:refnum<vi>, error out=w394:errorcluster)
          n176 = case shown="0, 1, 3" w400 {
            tunnel: w399 -> [_ w405]
            tunnel: w396 -> [_ w404]
            tunnel: w394 -> [w401 w403]
            tunnel: [w401 w402] -> w393
            frame 2, Default {
            }
            frame 0, 1, 3 {
              n177 = property class="Arr"(reference=w405, error in=w403, "Index Values"=w404) -> (error out=w402:errorcluster)  [unwired: 1 out]
            }
          }
        }
      }
      event "Component Name 10": Mouse Down; "Component Name 10": Mouse Up; "Component Name 10": Mouse Wheel {
        w416 = refnum<vi> refnum  # Array
        n178 = event-data() -> ("CtlRef"=w413:refnum<vi>)  [unwired: 1 in, 5 out]
        n179 = property on="Tab Control" class="TabCtl (strict)"(error in=w415) -> (error out=w412:errorcluster, "Pages"=w414:refnum<vi>[], "Value"=w409:T2)  [unwired: 1 in, 1 out]
        n180 = Index Array(array=w414, index=w409) -> (element=w411:refnum<vi>)
        n181 = property class="Arr (strict)"(reference=w413, error in=w412) -> (error out=w410:errorcluster, "Index Values"=w406:u32[])  [unwired: 1 out]
        n182 = property class="Page"(reference=w411, error in=w410) -> (error out=w408:errorcluster, "ControlsOnPage"=w417:refnum<vi>[])  [unwired: 1 out]
        n183 = for {
          tunnel: w417 -> [w423] mode=indexing
          tunnel: w416 -> [w422]
          tunnel: w406 -> [w421]
          shift-right: [w418] -> w407
          shift-left: w408 -> [w420]
          i -> [w425]
          n184 = To More Specific Class(target class=w422, reference=w423, error in=w420) -> (specific class reference=w424:refnum<vi>, error out=w419:errorcluster)
          n185 = case shown="0, 1, 3" w425 {
            tunnel: w424 -> [_ w430]
            tunnel: w421 -> [_ w429]
            tunnel: w419 -> [w426 w428]
            tunnel: [w426 w427] -> w418
            frame 2, Default {
            }
            frame 0, 1, 3 {
              n186 = property class="Arr"(reference=w430, error in=w428, "Index Values"=w429) -> (error out=w427:errorcluster)  [unwired: 1 out]
            }
          }
        }
      }
    }
  }
  n187 = while {
    shift-right: [w452] -> w57
    shift-left: w61 -> [w456]
    shift-right: [w432] -> w20
    shift-left: w29 -> [w458]
    tunnel: w10 -> [w450]
    shift-right: [w449] -> _
    shift-left: refnum<k34> refnum ("tdms file out") -> [w448]
    shift-right: [w447] -> _
    shift-left: w59 -> [w446]
    tunnel: w55 -> [w445]
    shift-right: [w442] -> _
    shift-left: _ -> [w441]
    shift-right: [w440] -> _
    shift-left: i32[][] [] ("Index Array") -> [w439]
    shift-right: [w438] -> _
    shift-left: string[] [] -> [w437]
    tunnel: w1 -> [w436]
    shift-right: [w435] -> _
    shift-left: _ -> [w434]
    stop <- w431 stop-if-true
    n188 = Dequeue Element(queue=w456, error in (no error)=w458) -> (queue out=w453:refnum<queue>, element=w457:T4, error out=w451:errorcluster)  [unwired: 1 in, 1 out]
    n189 = Unbundle By Name(w457) -> ("state"=w455:T1, "data"=w454:variant)
    "Internal State" <- w455
    n190 = Wait (ms)(milliseconds to wait=u32 100) -> ()  [unwired: 1 out]
    n191 = case shown="\"Initialize 2\"" w455 {
      tunnel: w454 -> [_ _ _ _ _ w627 _ _ w752 _ _ _ _ _ _ _ _ _ _ w1038 _ _]
      tunnel: w453 -> [w486 w510 w544 w575 w591 w626 w680 w727 w751 w759 w781 w797 w838 w866 w900 w934 w947 w970 w1002 w1045 w1103 w1115]
      tunnel: [w485 w509 w544 w574 w600 w618 w679 w714 w743 w757 w780 w794 w837 w865 w900 w933 w947 w969 w1001 w1045 w1102 w1114] -> w452
      tunnel: w451 -> [w484 w498 w543 w557 w590 w620 w676 w715 w745 w765 w778 w792 w836 w857 w894 w932 w952 w968 w984 w1039 w1098 w1121]
      tunnel: [w477 w494 w543 w572 w601 w625 w678 w713 w750 w758 w779 w795 w846 w864 w894 w905 w948 w967 w1000 w1021 w1101 w1120] -> w432
      tunnel: [w480 w493 w545 w573 w604 w622 w684 w726 w747 w766 w786 w804 w845 w878 w897 w930 TRUE w978 w999 w1042 w1104 w1119] -> w433
      tunnel: w450 -> [w468 _ _ w550 _ _ _ _ _ _ _ _ w833 w851 _ _ _ _ _ _ _ _]
      tunnel: [w488 w512 w547 w576 w605 w624 w686 w696 w749 w767 w785 w806 w847 w869 w899 w936 w959 w977 w1004 w1044 w1106 w1123] -> w449
      tunnel: w448 -> [w488 w512 w547 w576 w605 w624 w686 _ w749 w767 w785 w806 w847 w869 w899 w936 w959 w977 w1004 w1044 w1106 w1123]
      tunnel: [w487 w511 w546 w577 w593 w623 w685 w693 w748 w763 w784 w805 w848 w879 w898 w935 w953 w976 w1003 w1043 w1105 w1122] -> w447
      tunnel: w446 -> [w487 w511 w546 w577 w593 w623 w685 _ w748 w763 w784 w805 w848 w879 w898 w935 w953 w976 w1003 w1043 w1105 w1122]
      tunnel: w445 -> [_ w499 _ _ _ _ _ _ _ _ _ _ _ _ _ w931 _ _ _ _ _ _]
      tunnel: FALSE -> [w480 w493 w545 w573 w604 w622 w684 w726 w747 w766 w786 w804 w845 w878 w897 w930 _ w978 w999 w1042 w1104 w1119]
      tunnel: [w474 w492 w542 w565 w584 w609 w683 w725 w735 w764 w782 w803 w844 w877 w896 w904 w946 w975 w998 w1024 w1097 w1118] -> w442
      tunnel: w441 -> [w474 w492 w542 w565 _ w609 w683 w725 w735 w764 w782 w803 w844 w877 w896 w904 w946 w975 w998 w1024 w1097 w1118]
      tunnel: [w473 w491 w541 w564 w589 w608 w674 w695 w734 w762 w783 w802 w843 w876 w895 w903 w945 w974 w997 w1041 w1096 w1117] -> w440
      tunnel: w439 -> [w473 w491 w541 w564 w589 w608 w674 w695 _ w762 w783 w802 w843 w876 w895 w903 w945 w974 w997 w1041 w1096 w1117]
      tunnel: [w472 w490 w540 w563 w583 w607 w673 w692 w733 w754 w777 w791 w839 w862 w893 w902 w944 w973 w996 w1040 w1095 w1112] -> w438
      tunnel: w437 -> [w472 w490 w540 w563 w583 w607 w673 w692 w733 _ w777 w791 w839 w862 w893 w902 w944 w973 w996 w1040 w1095 w1112]
      tunnel: w436 -> [_ _ _ w552 _ _ _ _ _ _ _ _ w829 w850 _ _ _ _ _ _ _ _]
      tunnel: [w459 w489 w539 w551 w582 w606 w672 w691 w732 w753 w773 w787 w826 w849 w892 w901 w943 w965 w981 w1023 w1094 w1111] -> w435
      tunnel: w434 -> [w459 w489 w539 w551 w582 _ w672 w691 w732 w753 w773 w787 w826 w849 w892 w901 w943 w965 w981 w1023 w1094 w1111]
      frame "Run" {
        w470 = FALSE ("Independent Label")
        n192 = control-ref of="Register"() -> (w467:refnum<vi>)
        n193 = Build Array (concatenate)(w468, w467) -> (w466:refnum<vi>[])
        n194 = Enqueue Element(queue=w486, element=T4 {"state"=enum."Read ini file", "data"=variant} ("Cluster"), error in (no error)=w484) -> (queue out=w485:refnum<queue>, error out=w465:errorcluster)  [unwired: 1 in, 1 out]
        n195 = control-ref of="Run"() -> (w482:refnum<vi>)
        n196 = control-ref of="Exit"() -> (w471:refnum<vi>)
        n197 = call "Control Enable.vi"("error in (no error)"=w465, "Enum"=enum16{"Enb", "Dis", "Dis&G"}."Dis&G", "Reference Array"=w466) -> ("error out"=w462:errorcluster)  [unwired: 8 in]
        n198 = Build Array(w482, w471) -> (w463:refnum<vi>[])
        n199 = call "Control Enable.vi"("error in (no error)"=w462, "Enum"=enum16{"Enb", "Dis", "Dis&G"}."Enb", "Reference Array"=w463) -> ("error out"=w460:errorcluster)  [unwired: 8 in]
        n200 = property on="Status bar" class="Str"(error in=w460, "Value"="M100: Choose the correct paths for CSV and TDMS files; then, click Run." ("Status bar")) -> (error out=w479:errorcluster)  [unwired: 1 in, 1 out]
        n201 = property on="Tab Control" class="TabCtl (strict)"(error in=w479) -> (error out=w478:errorcluster, "Pages"=w476:refnum<vi>[])  [unwired: 1 in, 1 out]
        n202 = Reverse 1D Array(array=w476) -> (reversed array=w475:refnum<vi>[])
        n203 = call "Initialize Tab Control.vi"("Page Visible"=w470, "Independent Label"=w470, "error in"=w478, "Only clear"=FALSE, "Array"=w475) -> ("error out"=w477:errorcluster)  [unwired: 6 in]
      }
      frame "Read ini file" {
        n204 = Enqueue Element(queue=w510, element=T4 {"state"=enum."Idle", "data"=variant} ("Cluster"), error in (no error)=w498) -> (queue out=w509:refnum<queue>, error out=w496:errorcluster)  [unwired: 1 in, 1 out]
        n205 = Current VI's Path() -> (path=w502:path)
        n206 = disable-structure shown="Default" {
          disable-tunnel: w502 -> [w534 w538]
          disable-tunnel: [w533 w535] -> w501
          frame condition #0 (active) {
            n207 = Strip Path(path=w534) -> (stripped path=w533:path)  [unwired: 1 out]
          }
          frame condition #1 {
            n208 = Strip Path(path=w538) -> (stripped path=w537:path)  [unwired: 1 out]
            n209 = Strip Path(path=w537) -> (stripped path=w536:path)  [unwired: 1 out]
            n210 = Strip Path(path=w536) -> (stripped path=w535:path)  [unwired: 1 out]
          }
        }
        n211 = Build Path(base path=w501, name or relative path=w499) -> (appended path=w508:path)
        n212 = call <vilib>:"Open Config Data.vi"("error in (no error)"=w496, "create file if necessary (T)"=TRUE, "configuration file path"=w508) -> ("error out"=w506:errorcluster, "file created?"=w495:bool, "refnum"=w507:T9)  [unwired: 6 in]
        n213 = case shown="False" w495 {
          tunnel: w507 -> [w531 _]
          tunnel: w506 -> [w530 w532]
          tunnel: "csv config file" ("key") -> [w529 _]
          tunnel: "tdms file" ("key") -> [w527 _]
          tunnel: "version sheet" ("key") -> [w525 _]
          tunnel: [w522 w532] -> w494
          frame False {
            w523 = "Path" ("section")
            n214 = call-poly <vilib>:"Read Key.vi"("section"=w523, "error in (no error)"=w530, "key"=w529, "refnum"=w531) -> ("error out"=w515:errorcluster, "value"=w514:path, "refnum out"=w528:T9)  [unwired: 4 in, 1 out]
            n215 = property on="Config Path" class="Path"(error in=w515, "Value"=w514) -> (error out=w516:errorcluster)  [unwired: 1 in, 1 out]
            n216 = call-poly <vilib>:"Read Key.vi"("section"=w523, "error in (no error)"=w516, "key"=w527, "refnum"=w528) -> ("error out"=w518:errorcluster, "value"=w517:path, "refnum out"=w526:T9)  [unwired: 4 in, 1 out]
            n217 = property on="tdms path" class="Path"(error in=w518, "Value"=w517) -> (error out=w519:errorcluster)  [unwired: 1 in, 1 out]
            n218 = call-poly <vilib>:"Read Key.vi"("section"=w523, "error in (no error)"=w519, "key"=w525, "refnum"=w526) -> ("error out"=w520:errorcluster, "value"=w513:path, "refnum out"=w524:T9)  [unwired: 4 in, 1 out]
            n219 = property on="variation sheet" class="Path"(error in=w520, "Value"=w513) -> (error out=w521:errorcluster)  [unwired: 1 in, 1 out]
            n220 = call <vilib>:"Close Config Data.vi"("error in (no error)"=w521, "refnum"=w524) -> ("error out"=w522:errorcluster)  [unwired: 8 in, 1 out]
          }
          frame True {
          }
        }
      }
      frame "Idle", Default {
      }
      frame "Initialize 1" {
        w559 = TRUE ("Independent Label")
        n221 = control-ref of="Register"() -> (w548:refnum<vi>)
        n222 = Build Array (concatenate)(w550, w548) -> (w549:refnum<vi>[])
        n223 = call "Control Enable.vi"("error in (no error)"=w557, "Enum"=enum16{"Enb", "Dis", "Dis&G"}."Dis&G", "Reference Array"=w549) -> ("error out"=w555:errorcluster)  [unwired: 8 in]
        n224 = call "Control Enable.vi"("error in (no error)"=w555, "Enum"=enum16{"Enb", "Dis", "Dis&G"}."Enb", "Reference Array"=w552) -> ("error out"=w553:errorcluster)  [unwired: 8 in]
        n225 = property on="Tab Control" class="TabCtl (strict)"(error in=w553) -> (error out=w562:errorcluster, "Pages"=w561:refnum<vi>[])  [unwired: 1 in, 1 out]
        n226 = call "Initialize Tab Control.vi"("Page Visible"=w559, "Independent Label"=w559, "error in"=w562, "Only clear"=TRUE, "Array"=w561) -> ("error out"=w560:errorcluster)  [unwired: 6 in]
        n227 = property on="Status bar" class="Str"(error in=w560, "Value"="M200: The page was initialized by the latest configuration." ("Status bar")) -> (error out=w568:errorcluster)  [unwired: 1 in, 1 out]
        n228 = call <vilib>:"Is Path and Not Empty.vi"("path"="Config Path") -> ("Is Path and Not Empty?"=w569:bool)  [unwired: 4 in]
        n229 = case shown="True" w569 {
          tunnel: w568 -> [w578 w580]
          tunnel: [T4 {"state"=enum."Config file Error", "data"=variant} ("Cluster") T4 {"state"=enum."Read config file", "data"=variant} ("Cluster")] -> w567
          tunnel: [w578 w580] -> w566
          frame False {
          }
          frame True {
          }
        }
        n230 = Enqueue Element(queue=w575, element=w567, error in (no error)=w566) -> (queue out=w574:refnum<queue>, error out=w572:errorcluster)  [unwired: 1 in, 1 out]
      }
      frame "Read config file" {
        n231 = property on="Config Path" class="Path"(error in=w590) -> (error out=w599:errorcluster, "Value"=w602:path)  [unwired: 1 in, 1 out]
        n232 = call-poly <vilib>:"Read From Spreadsheet File.vi"("delimiter (\\t)"=";" ("delimiter (\\t)"), "transpose (no:F)"=FALSE, "file path (dialog if empty)"=w602) -> ("first row"=w588:string[], "all rows"=w594:string[][])  [unwired: 4 in, 3 out]
        n233 = property on="Tab Control" class="TabCtl (strict)"(error in=w599) -> (error out=w592:errorcluster, "Pages"=w586:refnum<vi>[])  [unwired: 1 in, 1 out]
        n234 = Array Size(array=w588) -> (size(s)=w587:i32)
        n235 = Array Subset(array=w586, index=0, length=w587) -> (w584:refnum<vi>[])
        n236 = To Variant(anything=w594) -> (Variant=w596:variant)
        n237 = Bundle By Name(cluster=T4 {"state"=enum."Update Comp Names", "data"=variant} ("Cluster"), "data"=w596) -> (w595:T4)
        n238 = Enqueue Element(queue=w591, element=w595, error in (no error)=w592) -> (queue out=w600:refnum<queue>, error out=w601:errorcluster)  [unwired: 1 in, 1 out]
      }
      frame "Update Comp Names" {
        n239 = Variant To Data(error in=w620, type=string[][] [] ("first row"), Variant=w627) -> (data=w619:string[][], error out=w616:errorcluster)
        n240 = Transpose 2D Array(2D array=w619) -> (transposed array=w613:string[][])
        n241 = for {
          shift-right: [w640] -> w612
          shift-left: w616 -> [w645]
          tunnel: w613 -> [w644] mode=indexing
          tunnel: [w638] -> w606 mode=indexing
          tunnel: w609 -> [w636] mode=indexing
          n242 = for {
            tunnel: w644 -> [w650] mode=indexing
            shift-right: [w651] -> w641
            shift-left: w645 -> [w652]
            shift-right: [w647] -> w639
            shift-left: string[] [] ("first row") -> [w648]
            tunnel: [w646] -> w642
            i -> [w646]
            stop <- w649 stop-if-true
            n243 = Equal To 0?(x=w646) -> (x = 0?=w653:bool)
            n244 = case shown="False" w653 {
              tunnel: w652 -> [w654 w671]
              tunnel: [w655 w671] -> w651
              tunnel: w650 -> [w658 _]
              tunnel: [w659 FALSE] -> w649
              tunnel: w648 -> [w657 w669]
              tunnel: [w656 w669] -> w647
              frame False {
                n245 = Empty String/Path?(string/path=w658) -> (empty?=w660:bool)
                n246 = case shown="False" w660 {
                  selector: w660 -> [w662 w668]
                  tunnel: [w662 w668] -> w659
                  tunnel: w658 -> [w664 _]
                  tunnel: w657 -> [w665 w667]
                  tunnel: [w663 w667] -> w656
                  tunnel: [w661 w666] -> w655
                  tunnel: w654 -> [w661 w666]
                  frame False {
                    n247 = Build Array (concatenate)(w665, w664) -> (w663:string[])
                  }
                  frame True {
                  }
                }
              }
              frame True {
              }
            }
          }
          n248 = Decrement(x=w642) -> (x-1=w638:i32)
          n249 = call "Values on Tab Ctrl.vi"("Max row"=12, "Tab page Refnum"=w636, "Error In"=w641, "no. Rows"=w638, "Value"=w639) -> ("Error Out"=w640:errorcluster)  [unwired: 6 in]
        }
        n250 = Index Array(array=w613, index (col)=0 ("disabled index (col)")) -> (element=w614:string[])  [unwired: 1 in]
        n251 = for {
          tunnel: w614 -> [w629] mode=indexing
          tunnel: w606 -> [w635] mode=indexing
          tunnel: [w628] -> w611 mode=indexing
          n252 = Number To Decimal String(number=w635, width (-)=i16 1) -> (decimal integer string=w632:string)
          n253 = Concatenate Strings(w629, " " ("string"), "(" ("string"), w632, ")" ("string")) -> (w628:string)
        }
        n254 = call "Update Tab Page Caption.vi"("error in"=w612, "Caption"=w611, "Pages ref"=w609) -> ("error out"=w610:errorcluster)  [unwired: 7 in, 1 out]
        n255 = Enqueue Element(queue=w626, element=T4 {"state"=enum."Initialize 2", "data"=variant} ("Cluster"), error in (no error)=w610) -> (queue out=w618:refnum<queue>, error out=w625:errorcluster)  [unwired: 1 in, 1 out]
      }
      frame "Initialize 2" {
        n256 = call <vilib>:"Is Path and Not Empty.vi"("path"="tdms path") -> ("Is Path and Not Empty?"=w682:bool)  [unwired: 4 in]
        n257 = case shown="True" w682 {
          tunnel: w676 -> [w687 w689]
          tunnel: [T4 {"state"=enum."Config file Error", "data"=variant} ("Cluster") T4 {"state"=enum."Read TDMS", "data"=variant} ("Cluster")] -> w677
          tunnel: [w687 w689] -> w675
          frame False {
          }
          frame True {
          }
        }
        n258 = Enqueue Element(queue=w680, element=w677, error in (no error)=w675) -> (queue out=w679:refnum<queue>, error out=w678:errorcluster)  [unwired: 1 in, 1 out]
      }
      frame "Read TDMS" {
        w698 = string[] []
        n259 = property on="tdms path" class="Path"(error in=w715) -> (error out=w711:errorcluster, "Value"=w712:path)  [unwired: 1 in, 1 out]
        n260 = TDMS Open(8:w711, 11:w712) -> (0:w724:errorcluster, 3:w723:refnum<k34>)  [unwired: 5 in]
        n261 = TDMS List Contents(4:w724, 6:"Version History" ("group name in (Untitled)"), 7:w723) -> (0:w710:errorcluster, 1:w707:string[], 2:w708:string, 3:w720:refnum<k34>)
        n262 = Reverse 1D Array(array=w707) -> (reversed array=w722:string[])
        n263 = Index Array(array=w722, index=0) -> (element=w706:string)
        n264 = TDMS Read(0:w720, 5:w708, 7:w706, 11:w710, 12:w698) -> (4:w701:refnum<k34>, 6:w700:string, 10:w718:string[], 15:w702:errorcluster)  [unwired: 3 in, 2 out]
        n265 = Array Size(array=w707) -> (size(s)=w719:i32)
        n266 = case shown="2, Default" w719 {
          tunnel: w718 -> [w728 w730]
          tunnel: [w728 w729] -> w717
          frame 2, Default {
          }
          frame 1 {
            n267 = for {
              tunnel: w730 -> [_] mode=indexing
              tunnel: ["no records!"] -> w729 mode=indexing
            }
          }
        }
        n268 = TDMS Read(0:w701, 5:w700, 7:"Component Name" ("group name in (Untitled)"), 11:w702, 12:w698) -> (4:w696:refnum<k34>, 10:w694:string[], 15:w697:errorcluster)  [unwired: 3 in, 3 out]
        n269 = Array Size(array=w694) -> (size(s)=w693:i32)
        n270 = Bundle(w717, w694) -> (w716:cluster{string[], string[]})  [unwired: 1 in]
        n271 = To Variant(anything=w716) -> (Variant=w703:variant)
        n272 = Bundle By Name(cluster=T4 {"state"=enum."Update Current Versions", "data"=variant} ("Cluster"), "data"=w703) -> (w705:T4)
        n273 = Enqueue Element(queue=w727, element=w705, error in (no error)=w697) -> (queue out=w714:refnum<queue>, error out=w713:errorcluster)  [unwired: 1 in, 1 out]
      }
      frame "Update Current Versions" {
        # "map component names in tabs to the component names in the TDMS file"
        n274 = Variant To Data(error in=w745, type=T7 {"Current Version"=[], "Comp Name"=[]} ("output cluster"), Variant=w752) -> (data=w746:T7, error out=w741:errorcluster)
        n275 = Unbundle By Name(w746) -> ("Current Version"=w736:string[], "Comp Name"=w740:string[])
        n276 = call "Index Component Names.vi"("Error In"=w741, "Comp Name"=w740, "Tab Page Ref"=w735) -> ("Error Out"=w739:errorcluster, "Index Array"=w734:i32[][], "Tab Page Ref dup"=w737:refnum<vi>[])  [unwired: 6 in]
        n277 = call "Update Current Versions.vi"("Error In"=w739, "Index Array"=w734, "Current Version"=w736, "Tab Page Ref"=w737) -> ("Error Out"=w738:errorcluster)  [unwired: 7 in]
        n278 = Enqueue Element(queue=w751, element=T4 {"state"=enum."Idle", "data"=variant} ("Cluster"), error in (no error)=w738) -> (queue out=w743:refnum<queue>, error out=w750:errorcluster)  [unwired: 1 in, 1 out]
      }
      frame "Make new configuration" {
        n279 = call "Make Configuration Array.vi"("Error In"=w765, "Number of components"=w763, "Index Array"=w762, "Tab Page Ref"=w764) -> ("Error Out"=w755:errorcluster, "no. Updates"=w761:u32, "New Configuration"=w754:string[])  [unwired: 4 in, 1 out]
        n280 = Greater Than 0?(x=w761) -> (x > 0?=w760:bool)
        n281 = case shown="True" w760 {
          tunnel: [T4 {"state"=enum."No New Update", "data"=variant} ("Cluster") T4 {"state"=enum."Update New Config", "data"=variant} ("Cluster")] -> w756
          frame False {
          }
          frame True {
          }
        }
        n282 = Enqueue Element(queue=w759, element=w756, error in (no error)=w755) -> (queue out=w757:refnum<queue>, error out=w758:errorcluster)  [unwired: 1 in, 1 out]
      }
      frame "Update New Config" {
        n283 = call "Update New Versions.vi"("Error In"=w778, "Index Array"=w783, "New Version"=w777, "Tab Page Ref"=w782) -> ("Error Out"=w775:errorcluster)  [unwired: 6 in, 1 out]
        n284 = property on="Register" class="Bool"(error in=w775, "DisabledEnum"=T8."Enabled" ("Disabled")) -> (error out=w772:errorcluster)  [unwired: 1 in, 1 out]
        n285 = property on="Status bar" class="Str"(error in=w772, "Val(Sgnl)"="M900: Configuration built. Ready to be registered. If any change is made, build config again." ("Value (Signaling)")) -> (error out=w771:errorcluster)  [unwired: 1 in, 1 out]
        n286 = Enqueue Element(queue=w781, element=T4 {"state"=enum."Idle", "data"=variant} ("Cluster"), error in (no error)=w771) -> (queue out=w780:refnum<queue>, error out=w779:errorcluster)  [unwired: 1 in, 1 out]
      }
      frame "Register Change" {
        n287 = call "Confirm changes"("error in (no error)"=w792) -> ("Sign with your name"=w798:string, "Confirm"=w799:bool, "error out"=w800:errorcluster)  [unwired: 16 in]
        n288 = case shown="True" w799 {
          tunnel: w806 -> [_ w821]
          tunnel: w800 -> [w808 w816]
          tunnel: w791 -> [_ w813]
          tunnel: w797 -> [w807 w812]
          tunnel: ["M400: The configuration was rejected." ("F button name (\"Cancel\")") "M300: The configuration was successfully registered. Refresh the page to continue." ("F button name (\"Cancel\")")] -> w801
          tunnel: w798 -> [_ w818]
          tunnel: [w808 w811] -> w790
          tunnel: [w807 w812] -> w793
          frame False {
          }
          frame True {
            n289 = Build Array(w818) -> (w817:string[])
            n290 = Get Date/Time In Seconds() -> (seconds since 1Jan1904=w823:timestamp)
            n291 = Format Date/Time String(time format string (%c)="Date: %Y-%b-%d    Time: %H:%M:%S", seconds (now)=w823) -> (date/time string=w819:string)  [unwired: 1 in]
            n292 = TDMS Write(0:w821, 5:"Reporter" ("group name in (Untitled)"), 7:w819, 9:w817, 11:w816) -> (4:w815:refnum<k34>, 8:w814:string, 15:w822:errorcluster)  [unwired: 1 in, 1 out]
            n293 = TDMS Write(0:w815, 5:"Version History" ("group name in (Untitled)"), 7:w814, 9:w813, 11:w822) -> (15:w811:errorcluster)  [unwired: 1 in, 3 out]
          }
        }
        "Status bar" <- w801
        n294 = property on="Register" class="Bool"(error in=w790, "DisabledEnum"=T8."Disabled and Grayed Out" ("Disabled")) -> (error out=w789:errorcluster)  [unwired: 1 in, 1 out]
        n295 = Enqueue Element(queue=w793, element=T4 {"state"=enum."Idle", "data"=variant} ("Cluster"), error in (no error)=w789) -> (queue out=w794:refnum<queue>, error out=w795:errorcluster)  [unwired: 1 in, 1 out]
      }
      frame "View Registry" {
        n296 = property on="Status bar" class="Str"(error in=w836, "Value"="M1000: View the registry." ("Status bar")) -> (error out=w834:errorcluster)  [unwired: 1 in, 1 out]
        n297 = call "Control Enable.vi"("error in (no error)"=w834, "Enum"=enum16{"Enb", "Dis", "Dis&G"}."Dis&G", "Reference Array"=w833) -> ("error out"=w831:errorcluster)  [unwired: 8 in]
        n298 = property on="tdms path" class="Path"(error in=w831) -> (error out=w841:errorcluster, "Value"=w842:path)  [unwired: 1 in, 1 out]
        n299 = call <vilib>:"TDMS - File Viewer.vi"("error in (no error)"=w841, "file path"=w842) -> ("error out"=w830:errorcluster)  [unwired: 4 in, 1 out]
        n300 = call "Control Enable.vi"("error in (no error)"=w830, "Enum"=enum16{"Enb", "Dis", "Dis&G"}."Enb", "Reference Array"=w829) -> ("error out"=w827:errorcluster)  [unwired: 8 in]
        n301 = Enqueue Element(queue=w838, element=T4 {"state"=enum."Idle", "data"=variant} ("Cluster"), error in (no error)=w827) -> (queue out=w837:refnum<queue>, error out=w846:errorcluster)  [unwired: 1 in, 1 out]
      }
      frame "Add Comment" {
        n302 = call "Control Enable.vi"("error in (no error)"=w857, "Enum"=enum16{"Enb", "Dis", "Dis&G"}."Dis&G", "Reference Array"=w851) -> ("error out"=w856:errorcluster)  [unwired: 8 in]
        n303 = call "Add Comment.vi"("Error In"=w856) -> ("Error Out"=w861:errorcluster, "Comment out"=w860:string, "Commentor out"=w859:string, "Add?"=w858:bool)  [unwired: 7 in]
        n304 = Build Array(w859, w860) -> (w872:string[])
        n305 = TDMS List Contents(4:w861, 6:"Version History" ("group name in (Untitled)"), 7:w869) -> (0:w868:errorcluster, 1:w870:string[], 3:w875:refnum<k34>)  [unwired: 1 out]
        n306 = case shown="False" w858 {
          tunnel: w875 -> [_ w891]
          tunnel: [w881 w890] -> w874
          tunnel: w872 -> [_ w883]
          tunnel: "Comment" ("group name in (Untitled)") -> [_ w886]
          tunnel: w870 -> [_ w887]
          tunnel: w868 -> [w881 w885]
          tunnel: ["M501: Comment was rejected." ("Status bar") "M500: Comment was successfully added to the latest entry." ("Status bar")] -> w863
          frame False {
          }
          frame True {
            n307 = Reverse 1D Array(array=w887) -> (reversed array=w888:string[])
            n308 = Index Array(array=w888, index=0) -> (element=w882:string)
            n309 = TDMS Write(0:w891, 5:w886, 7:w882, 9:w883, 11:w885) -> (15:w890:errorcluster)  [unwired: 1 in, 3 out]
          }
        }
        n310 = property on="Status bar" class="Str"(error in=w874, "Value"=w863) -> (error out=w854:errorcluster)  [unwired: 1 in, 1 out]
        n311 = call "Control Enable.vi"("error in (no error)"=w854, "Enum"=enum16{"Enb", "Dis", "Dis&G"}."Enb", "Reference Array"=w850) -> ("error out"=w853:errorcluster)  [unwired: 8 in]
        n312 = Enqueue Element(queue=w866, element=T4 {"state"=enum."Idle", "data"=variant} ("Cluster"), error in (no error)=w853) -> (queue out=w865:refnum<queue>, error out=w864:errorcluster)  [unwired: 1 in, 1 out]
      }
      frame "Check current versions" {
      }
      frame "Write ini file" {
        w914 = "Path" ("section")
        n313 = Current VI's Path() -> (path=w921:path)
        n314 = disable-structure shown="RUN_TIME_ENGINE==True" {
          disable-tunnel: w921 -> [w938 w942]
          disable-tunnel: [w937 w939] -> w920
          frame condition #0 (active) {
            n315 = Strip Path(path=w938) -> (stripped path=w937:path)  [unwired: 1 out]
          }
          frame condition #1 {
            n316 = Strip Path(path=w942) -> (stripped path=w941:path)  [unwired: 1 out]
            n317 = Strip Path(path=w941) -> (stripped path=w940:path)  [unwired: 1 out]
            n318 = Strip Path(path=w940) -> (stripped path=w939:path)  [unwired: 1 out]
          }
        }
        n319 = Build Path(base path=w920, name or relative path=w931) -> (appended path=w929:path)
        n320 = call <vilib>:"Open Config Data.vi"("error in (no error)"=w932, "create file if necessary (T)"=FALSE, "configuration file path"=w929) -> ("error out"=w912:errorcluster, "refnum"=w928:T9)  [unwired: 6 in, 1 out]
        n321 = property on="Config Path" class="Path"(error in=w912) -> (error out=w911:errorcluster, "Value"=w923:path)  [unwired: 1 in, 1 out]
        n322 = call-poly <vilib>:"Write Key.vi"("section"=w914, "error in (no error)"=w911, "value"=w923, "key"="csv config file", "refnum"=w928) -> ("error out"=w910:errorcluster, "refnum out"=w926:T9)  [unwired: 4 in, 1 out]
        n323 = property on="tdms path" class="Path"(error in=w910) -> (error out=w909:errorcluster, "Value"=w922:path)  [unwired: 1 in, 1 out]
        n324 = call-poly <vilib>:"Write Key.vi"("section"=w914, "error in (no error)"=w909, "value"=w922, "key"="tdms file", "refnum"=w926) -> ("error out"=w908:errorcluster, "refnum out"=w919:T9)  [unwired: 4 in, 1 out]
        n325 = property on="variation sheet" class="Path"(error in=w908) -> (error out=w907:errorcluster, "Value"=w918:path)  [unwired: 1 in, 1 out]
        n326 = call-poly <vilib>:"Write Key.vi"("section"=w914, "error in (no error)"=w907, "value"=w918, "key"="version sheet", "refnum"=w919) -> ("error out"=w916:errorcluster, "refnum out"=w915:T9)  [unwired: 4 in, 1 out]
        n327 = call <vilib>:"Close Config Data.vi"("error in (no error)"=w916, "refnum"=w915) -> ("error out"=w906:errorcluster)  [unwired: 8 in, 1 out]
        n328 = Enqueue Element(queue=w934, element=T4 {"state"=enum."Close", "data"=variant} ("Cluster"), error in (no error)=w906) -> (queue out=w933:refnum<queue>, error out=w905:errorcluster)  [unwired: 1 in, 1 out]
      }
      frame "Close" {
        n329 = Release Queue(queue=w947, error in (no error)=w952) -> (error out=w951:errorcluster)  [unwired: 1 in, 2 out]
        n330 = TDMS Close(8:w951, 11:w959) -> (0:w950:errorcluster)  [unwired: 1 out]
        n331 = control-ref of="Run"() -> (w958:refnum<vi>)
        n332 = property class="Bool"(reference=w958, error in=w950, "DisabledEnum"=T8."Enabled" ("Disabled")) -> (error out=w956:errorcluster)  [unwired: 1 out]
        n333 = property on="Status bar" class="Str"(error in=w956, "Value"="M700: Application terminated." ("Status bar")) -> (error out=w949:errorcluster)  [unwired: 1 in, 1 out]
        n334 = disable-structure shown="RUN_TIME_ENGINE==True" {
          disable-tunnel: w949 -> [w961 w964]
          disable-tunnel: [w961 w964] -> w948
          disable-tunnel: TRUE ("quit? (T)") -> [w962 w963]
          frame condition #0 (active) {
            n335 = Stop(stop? (T)=w962) -> ()
          }
          frame condition #1 {
            n336 = Quit LabVIEW(quit? (T)=w963) -> ()
          }
        }
      }
      frame "Check ini file" {
        n337 = call <vilib>:"Is Path and Not Empty.vi"("path"="variation sheet") -> ("Is Path and Not Empty?"=w971:bool)  [unwired: 4 in]
        n338 = case shown="True" w971 {
          tunnel: [T4 {"state"=enum."Config file Error", "data"=variant} ("Cluster") T4 {"state"=enum."Read Variation Sheet", "data"=variant} ("Cluster")] -> w966
          frame False {
          }
          frame True {
          }
        }
        n339 = Enqueue Element(queue=w970, element=w966, error in (no error)=w968) -> (queue out=w969:refnum<queue>, error out=w967:errorcluster)  [unwired: 1 in, 1 out]
      }
      frame "Read Variation Sheet" {
        w988 = T4 {"state"=enum."Search and write current versions", "data"=variant}  # Cluster
        n340 = property on="variation sheet" class="Path"(error in=w984) -> (error out=w985:errorcluster, "Value"=w983:path)  [unwired: 1 in, 1 out]
        n341 = call <vilib>:"Open Config Data.vi"("error in (no error)"=w985, "create file if necessary (T)"=FALSE, "configuration file path"=w983) -> ("error out"=w994:errorcluster, "refnum"=w993:T9)  [unwired: 6 in, 1 out]
        n342 = call <vilib>:"Get Section Names.vi"("error in (no error)"=w994, "refnum"=w993) -> ("error out"=w992:errorcluster, "section names"=w990:string[], "refnum out"=w991:T9)  [unwired: 7 in]
        n343 = for {
          tunnel: w990 -> [w1007] mode=indexing
          shift-right: [w1006] -> w986
          shift-left: w992 -> [w1011]
          tunnel: w991 -> [w1012]
          tunnel: [w1005] -> w982 mode=indexing
          n344 = call <vilib>:"Get Key Names.vi"("section"=w1007, "error in (no error)"=w1011, "refnum"=w1012) -> ("error out"=w1008:errorcluster, "key names"=w1009:string[], "refnum out"=w1010:T9)  [unwired: 5 in, 1 out]
          n345 = for {
            tunnel: w1010 -> [w1020]
            tunnel: w1009 -> [w1014] mode=indexing
            shift-right: [w1018] -> w1006
            shift-left: w1008 -> [w1019]
            tunnel: w1007 -> [w1016]
            tunnel: [w1017] -> _ mode=indexing
            tunnel: [w1015] -> w1005 mode=indexing
            n346 = call-poly <vilib>:"Read Key.vi"("section"=w1016, "error in (no error)"=w1019, "key"=w1014, "refnum"=w1020) -> ("error out"=w1018:errorcluster, "value"=w1013:string, "refnum out"=w1017:T9)  [unwired: 4 in, 1 out]
            n347 = Build Array(w1016, w1014, w1013) -> (w1015:string[])
          }
        }
        n348 = To Variant(anything=w982) -> (Variant=w987:variant)
        n349 = Bundle By Name(cluster=w988, "data"=w987) -> (w989:T4)
        n350 = Enqueue Element(queue=w1002, element=w989, error in (no error)=w986) -> (queue out=w1001:refnum<queue>, error out=w1000:errorcluster)  [unwired: 1 in, 1 out]
      }
      frame "Search and write current versions" {
        n351 = Variant To Data(error in=w1039, type=string[][][] [], Variant=w1038) -> (data=w1033:string[][][], error out=w1028:errorcluster)
        n352 = property on="Config Path" class="Path"(error in=w1028) -> (error out=w1046:errorcluster, "Value"=w1031:path)  [unwired: 1 in, 1 out]
        n353 = Array Size(array=w1033) -> (size(s)=w1036:i32[])
        n354 = Index Array(array=w1036, index=0) -> (element=w1034:i32)
        n355 = call-poly <vilib>:"Read From Spreadsheet File.vi"("delimiter (\\t)"=";" ("delimiter (\\t)"), "transpose (no:F)"=FALSE, "file path (dialog if empty)"=w1031) -> ("all rows"=w1029:string[][])  [unwired: 4 in, 4 out]
        n356 = Transpose 2D Array(2D array=w1029) -> (transposed array=w1027:string[][])
        n357 = Index Array(array=w1027, index (col)=0 ("disabled index (col)")) -> (element=w1025:string[])  [unwired: 1 in]
        n358 = for {
          N: w1034 -> [_]
          tunnel: w1033 -> [w1061]
          tunnel: w1025 -> [w1057]
          tunnel: w1024 -> [w1054]
          shift-right: [w1051] -> w1022
          shift-left: w1046 -> [w1052]
          tunnel: w1023 -> [w1050]
          i -> [w1060]
          w1059 = 0 ("index (row)")
          n359 = Index Array(array=w1061, index (dim 0)=w1060) -> (element=w1053:string[][])  [unwired: 2 in]
          n360 = Index Array(array=w1053, index (row)=w1059, index (col)=w1059) -> (element=w1058:string)
          n361 = Search 1D Array(1D array=w1057, element=w1058, start index (0)=0) -> (index of element=w1055:i32)
          n362 = case shown="0, Default" w1055 {
            selector: w1055 -> [w1066 _]
            tunnel: w1054 -> [w1074 _]
            tunnel: w1053 -> [w1073 _]
            tunnel: w1052 -> [w1063 w1093]
            tunnel: [w1068 w1093] -> w1051
            tunnel: w1050 -> [w1067 _]
            frame 0, Default {
              n363 = Index Array(array=w1074, index=w1066) -> (element=w1065:refnum<vi>)
              n364 = Index Array(array=w1067, index=w1066) -> (element=w1064:i32)
              n365 = Index Array(array=w1073, index (col) #1=1 ("disabled index (col)"), index (col) #2=2 ("index (col)")) -> (element #1=w1071:string[], element #2=w1069:string[])  [unwired: 2 in]
              n366 = call "Initialize New Configuration Array.vi"("error in"=w1063, "no. elements"=w1064, "Page Refnum"=w1065) -> ("error out"=w1062:errorcluster)  [unwired: 7 in, 1 out]
              n367 = for {
                tunnel: w1071 -> [w1078] mode=indexing
                tunnel: w1065 -> [w1079]
                shift-right: [w1076] -> w1068
                shift-left: w1062 -> [w1077]
                tunnel: w1069 -> [w1075] mode=indexing
                stop <- w1080 stop-if-true
                n368 = Empty String/Path?(string/path=w1078) -> (empty?=w1081:bool)
                n369 = case shown="False" w1081 {
                  selector: w1081 -> [w1090 w1092]
                  tunnel: [w1090 w1092] -> w1080
                  tunnel: w1079 -> [w1089 _]
                  tunnel: w1078 -> [w1088 _]
                  tunnel: w1077 -> [w1087 w1091]
                  tunnel: [w1083 w1091] -> w1076
                  tunnel: w1075 -> [w1082 _]
                  frame False {
                    n370 = call "Search Component Name.vi"("error in"=w1087, "Element"=w1088, "Page Refnum"=w1089) -> ("error out"=w1086:errorcluster, "index of element"=w1084:i32, "Page Refnum"=w1085:refnum<vi>)  [unwired: 6 in]
                    n371 = call "Write Version from ini File.vi"("error in"=w1086, "Entry"=w1082, "index of element"=w1084, "Page Refnum"=w1085) -> ("error out"=w1083:errorcluster)  [unwired: 6 in, 1 out]
                  }
                  frame True {
                  }
                }
              }
            }
            frame -1 {
            }
          }
        }
        n372 = disable-structure shown="Disabled" {
          disable-tunnel: w1022 -> [w1049 _]
          disable-tunnel: [w1048 _] -> w1021
          frame Disabled {
            n373 = call "Control Enable.vi"("error in (no error)"=w1049, "Enum"=enum16{"Enb", "Dis", "Dis&G"}."Enb") -> ("error out"=w1048:errorcluster)  [unwired: 9 in]
          }
          frame Enabled {
          }
        }
      }
      frame "Config file Error" {
        n374 = One Button Dialog(message="Error in (csv, tdms, or ini) file path.\nEither Not A Path or Path is Empty.", button name ("OK")="Check File Paths") -> (true=w1099:bool)
        n375 = case shown="True" w1099 {
          tunnel: [T4 {"state"=enum."Idle", "data"=variant} ("Cluster") T4 {"state"=enum."Run", "data"=variant} ("Cluster")] -> w1100
          frame False {
          }
          frame True {
          }
        }
        n376 = Enqueue Element At Opposite End(queue=w1103, element=w1100, error in (no error)=w1098) -> (queue out=w1102:refnum<queue>, error out=w1101:errorcluster)  [unwired: 1 in, 1 out]
      }
      frame "No New Update" {
        n377 = flat-sequence {
          tunnel: w1121 -> [w1127]
          tunnel: [w1127] -> w1116
          tunnel: [w1124] -> _
          frame #0 {
            n378 = One Button Dialog(message="There is no new updates. To register a new configuration, you need at least one new version.\nThe page will be reinitialized with the latest configuration.", button name ("OK")="OK") -> (true=w1124:bool)
          }
        }
        n379 = Enqueue Element(queue=w1115, element=T4 {"state"=enum."Idle", "data"=variant} ("Cluster"), error in (no error)=w1116) -> (queue out=w1114:refnum<queue>, error out=w1120:errorcluster)  [unwired: 1 in, 1 out]
      }
    }
    n380 = Or(x=w432, y=w433) -> (x .or. y?=w431:bool)
  }
  n381 = Merge Errors(w20, w18) -> (w19:errorcluster)
  n382 = Release Queue(queue=w57, error in (no error)=w19) -> (error out=w56:errorcluster)  [unwired: 1 in, 2 out]
  n383 = call <vilib>:"Simple Error Handler.vi"("error in (no error)"=w56) -> ()  [unwired: 4 in, 5 out]
